vi "meb2cx_ver4_1_16bit.vi"() -> ()   [LabVIEW 2019]
uses:
  <vilib>/Analysis/3filter.llb/Filter Passband Type.ctl
  <vilib>/Utility/error.llb/DialogType.ctl
  <vilib>/DAQmx/write.llb/DAQmx Write (Analog 2D DBL NChan NSamp).vi
  <vilib>/DAQmx/read.llb/DAQmx Read (Analog 1D DBL 1Chan NSamp).vi
  <vilib>/DAQmx/read.llb/DAQmx Read (Analog 2D DBL NChan NSamp).vi
  <vilib>/Analysis/8numeric.llb/1D Numeric Integration.vi
  <vilib>/DAQmx/write.llb/DAQmx Write (Digital U16 1Chan 1Samp).vi
  <vilib>/DAQmx/read.llb/DAQmx Read (Analog DBL 1Chan 1Samp).vi
  <vilib>/Utility/file.llb/Read Delimited Spreadsheet (DBL).vi
  <vilib>/DAQmx/create/channels.llb/DAQmx Create Channel (DO-Digital Output).vi
  <vilib>/DAQmx/create/channels.llb/DAQmx Create Channel (AO-Voltage-Basic).vi
  <vilib>/DAQmx/create/channels.llb/DAQmx Create Channel (AI-Voltage-Basic).vi
  <vilib>/Analysis/3filter.llb/Butterworth Filter (DBL).vi
  <vilib>/DAQmx/configure/timing.llb/DAQmx Timing (Sample Clock).vi
  <vilib>/DAQmx/miscellaneous.llb/DAQmx Fill In Error Info.vi
  <vilib>/DAQmx/configure/trigger.llb/DAQmx Start Trigger (Digital Edge).vi
  <vilib>/Utility/file.llb/Write Delimited Spreadsheet (DBL).vi
  <vilib>/measure/madcrms.llb/Averaged DC-RMS for 1 Chan.vi
  <vilib>/measure/mascope.llb/Amplitude and Levels 1 chan.vi
  <vilib>/addons/Digital Filter Design/Process.llb/DFD Filtering (Array).vi
  <vilib>/Analysis/Matrix/Numeric/Conversions/Array To Matrix - RA2.vi
  <vilib>/Analysis/Matrix/Comparison/Equal/Equal - RM,RM.vi
  <vilib>/measure/NI_MAPro.lvlib
  <vilib>/Analysis/NI_AALPro.lvlib
  <vilib>/Analysis/NI_AAL_SigProc.lvlib
  <vilib>/Analysis/NI_AALBase.lvlib
  <resource>/objmgr/daqmx.rc
  <vilib>/gmath/NI_Gmath.lvlib
  <vilib>/addons/Digital Filter Design/NI_DigFilterLicensed.lvlib
  <vilib>/Analysis/Matrix/NI_Matrix.lvlib
panel:
  in  "stop delay":bool
  out "GERROR":bool
  out "error out 2":errorcluster
  out "error out":errorcluster
  out "CAL2":dbl[](array[numeric])
  out "YY":dbl[](array[numeric])
  out "XX":dbl[](array[numeric])
  out "F Si PSI":dbl format="%#.0f"
  out "bool_list":bool
  in  "Pomiar_main":bool
  out "Saveindi":bool=TRUE
  in  "Tab Control":enum32{"STAT", "MEAS", "CAL", "STOR", "TOOL"}(tab)
  out "Dev_Ready":bool
  out "Waveform Graph 5":dbl[][](graph)
  out "Bat_Low":bool
  out "Waveform Graph 4":dbl[][](graph)
  out "wz":u8[](array[numeric])=[0, 1, 2, 4, 5, 6, 8, 9, 10, 12, 13, 14, 28, 29, 30, 44, 45, 46, 60, 76, 77, 78, 92, 93, 94, 108, 109, 110, 124, 140, 141]
  in  "Gfreq":dbl=10.0 format="%0.4e"
  in  "stop":bool
  out "Supply [V]":dbl format="%#.1f"
  in  "Gain\n[dB]":u8 max=60 step=2
  in  "DEL":bool
  out "F Quality":dbl format="%#.0f"
  out "F Si":dbl format="%#.0f"
  in  "FREEZE":bool
  out "Si[MPa]":dbl max=200.0 format="%#.0f"
  out "Count":i32
  out "Waveform Graph 2":dbl[](graph)
  out "Low_L":dbl format="%.2g"
  out "Hi_L":dbl format="%.2g"
  out "AMP":dbl format="%.1f"
  out "INT":i32 format="%#.0f"
  out "XY Graph 2":cluster{"X":dbl, "Y":dbl}[](graph)
  in  "Oblicz":bool
  in  "SAVE":bool
  out "REC.":dbl
  out "Quality":i32
  out "F INT":dbl format="%#.0f"
  out "F Count":dbl
  out "F Amp":dbl format="%.1g"
  in  "AUTO":bool
  in  "Manual":bool
  in  "Delete cal file":bool
  out "Si [MPa]":dbl format="%#.0f"
  out "Int/Count":dbl format="%#.0f"
  out "cal3":dbl
  out "cal2":dbl
  out "cal1":dbl format="%#.0f"
  in  "OK cal3":bool
  in  "OK cal2":bool
  in  "OK cal1":bool
  out "XY Graph":cluster{"X":dbl, "Y":dbl}[](graph)
  in  "Load calibration":bool
  out "Quality":dbl format="%#.1f"
  in  "Calibration file to load":string(combo)
  in  "Import calibration files":bool
  out "cal4":dbl
  in  "OK cal4":bool
  in  "ListuDow":bool
  in  "Delete content":bool
  in  "Listbox":i32(listbox)=-1
  out "Active file":string
  out "Preview":dbl[](graph)
  in  "Save data file":bool
  in  "File load and\nexport source":string(combo)="A"
  in  "Export to drive":bool
  out "Export in\nprogress":bool
  in  "Preview data":bool
  in  "Delete folder content":bool
  in  "Plot selection":u16(ring) items=["AMP"=0, "INT"=3, "Count"=4, "Si[MPa]"=5, "Quality"=6]
  in  "ListUP":bool
  in  "FFT RANGE":i32 min=0
  in  "Update":bool
  in  "Set time":bool
  out "Waveform Graph 6":cluster{"rms_sign":dbl[]}[](graph)
  in  "filtrFFT":dbl=10.0 format="%0.2p"
  in  "filtrRMS":dbl=25.0 format="%0.2p"
  in  "THRESHOLD":dbl=1.7999999999999998 min=0.0 max=5.0 step=0.2
  in  "SOURCE":bool
  in  "FFT RANGE":cluster{"START":dbl, "END":dbl}[](array[cluster])
  out "XY Graph 3":cluster{"X":dbl, "Y":dbl}[](graph)
  out "Waveform Graph":cluster{"Filtered X":dbl[]}[](graph)
  in  "CF":dbl=5.000000000000002 min=0.0 max=10.0 step=0.2
  out "Waveform Graph 3":dbl[](graph)
  in  "Del_ZERO":bool
  in  "P_Zero":bool
  out "Boolean 8":bool
  out "Boolean 7":bool
  out "Boolean 6":bool
  out "Boolean 5":bool
  out "enUP":dbl format="%#.1g"
  out "Byłem":bool
  out "MPzero":dbl[][](array[numeric])
  out "Licznik":u8 max=60 step=2
  out "AAZero":dbl[][](array[numeric])
  out "P_Quality":i32
  out "TLO":dbl[](array[numeric])
  out "HBN_LOOP":dbl[](array[numeric])
  out "OK":bool
  out "Low_L 2":dbl format="%.2g"
  out "Hi_L 2":dbl format="%.2g"
  out "Data output":dbl[][](array[numeric])
  out "CAL":dbl[][](array[numeric])
  out "BAT":refnum<k21>
  out "ALL":dbl[][](array[numeric]) format="%0.2f"
  out "HBN":dbl[](array[numeric]) format="%0.2f"
  out "Trest":refnum<k21>
  out "Thbn":refnum<k21>
  out "Tgen":refnum<k21>
  out "Twz":refnum<k21>
  # "MAGSTRESS 5C - ser. 20200005"
  # "ver 4_1_16bit"
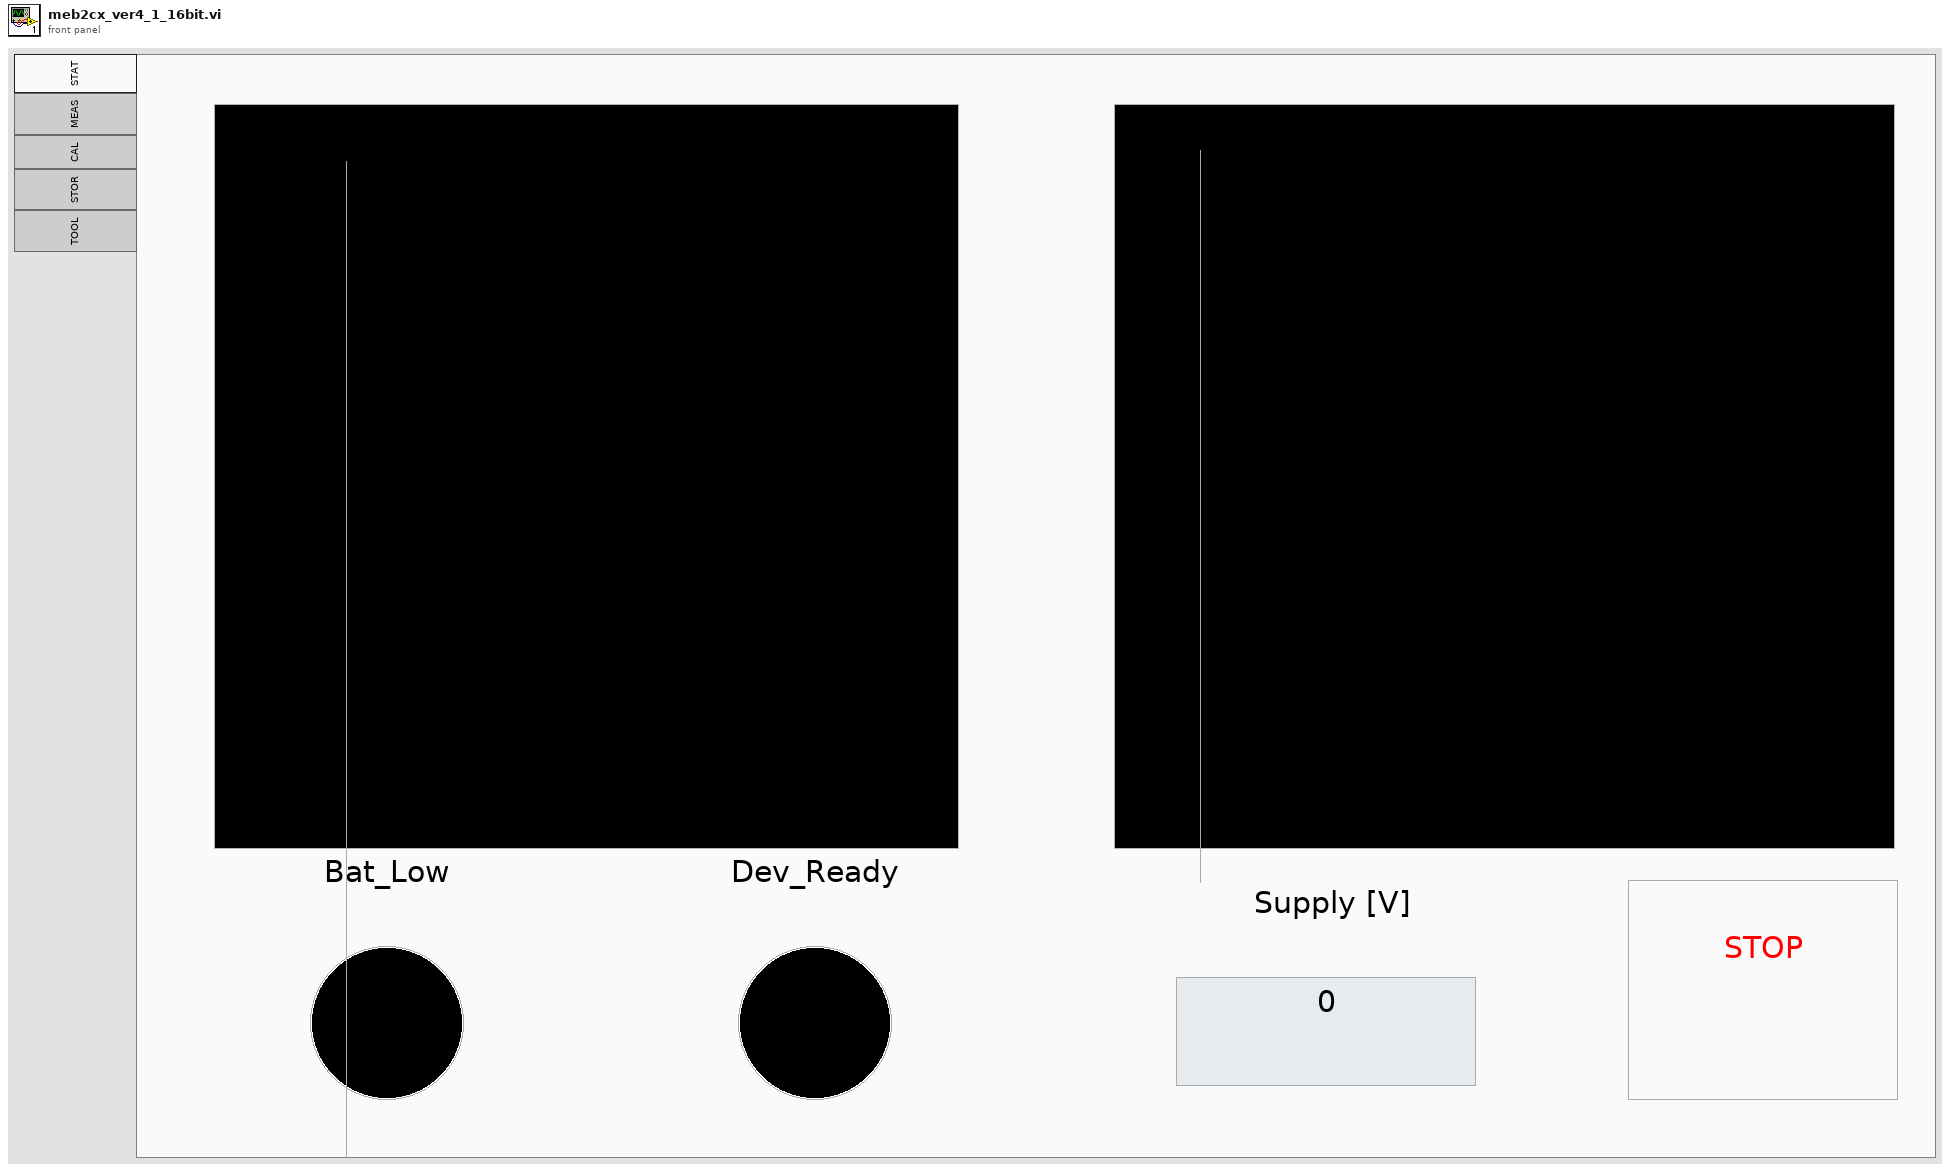
[diagram p1: front panel]
types:
  T1 = enum8{"Enabled", "Disabled", "Disabled and Grayed Out"}
  T2 = typedef "NI_AALBase.lvlib/Filter Passband Type.ctl" = enum32{"Lowpass", "Highpass", "Bandpass", "Bandstop"}
  T3 = typedef "DialogType.ctl" = u16
  T4 = typedef "NI_DigFilterLicensed.lvlib/DFD Filter Obj.ctl" = cluster{"mSRate_Fs":dbl, "mSRate_Version":string, "mSRate_Comments":string, "mSRate_OrgCoef":T5, "mSRate_CurCoef":T5, "mSRate_Quantized?":bool, "mSRate_QCoef":T5, "mSRate_QSettings":T7[], "mSRate_Order":i32, "mSRate_Scaling":cluster{"mSRate_ScaleByPowerOf2?":bool, "mSRate_ScaleType":T9}}
  T5 = typedef "NI_DigFilterLicensed.lvlib/DFD Filter Coef.ctl" = cluster{"type":T6, "gain":dbl, "coef a (k)":dbl[], "coef b (v)":dbl[]}
  T6 = typedef "NI_DigFilterLicensed.lvlib/DFD Filter Structure Type Selector.ctl" = enum16{"Undefined", "FIR Direct Form", "FIR Direct Form Transposed", "FIR Symmetric", "FIR Antisymmetric", "IIR Direct Form I", "IIR Direct Form I Transposed", "IIR Direct Form II", "IIR Direct Form II Transposed", "IIR Cascaded Second Order Sections Form I", "IIR Cascaded Second Order Sections Form I Transposed", "IIR Cascaded Second Order Sections Form II", "IIR Cascaded Second Order Sections Form II Transposed", "Lattice Allpass (basic sections)", "Lattice Allpass (one multiplier sections)", "Lattice Allpass (normalized sections)", "Lattice AR (basic sections)", "Lattice AR (one multiplier sections)", "Lattice AR (normalized sections)", "Lattice MA (minimum phase)", "Lattice MA (maximum phase)", "Lattice ARMA (basic sections)", "Lattice ARMA (one multiplier sections)", "Lattice ARMA (normalized sections)"}
  T7 = typedef "NI_DigFilterLicensed.lvlib/dfd_Internal Quantization Settings.ctl" = cluster{"source":T8, "wl":i16, "iwl":i16, "overflow mode":enum16{"Saturation", "Wrap"}, "rounding mode":enum16{"Nearest", "Truncation"}, "signed?":bool}
  T8 = typedef "NI_DigFilterLicensed.lvlib/dfd_Internal Quantization Srcs.ctl" = u16
  T9 = typedef "NI_DigFilterLicensed.lvlib/DFD Coef Norm Type.ctl" = enum16{"No Norm", "Time Domain 1-Norm", "Time Domain 2-Norm", "Time Domain Inf-Norm"}
  T10 = typedef "NI_Matrix.lvlib/RealMatrix.ctl" = dbl[][]
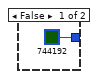
[diagram p3: hidden frame]
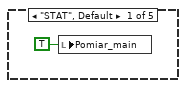
[diagram p4: hidden frame]
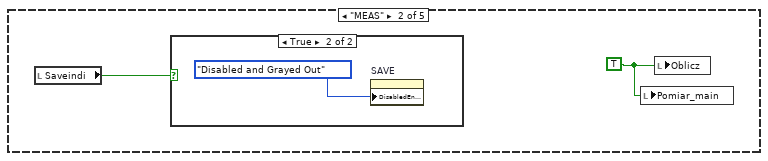
[diagram p5: hidden frame]
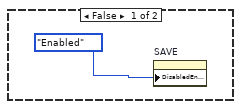
[diagram p6: hidden frame]
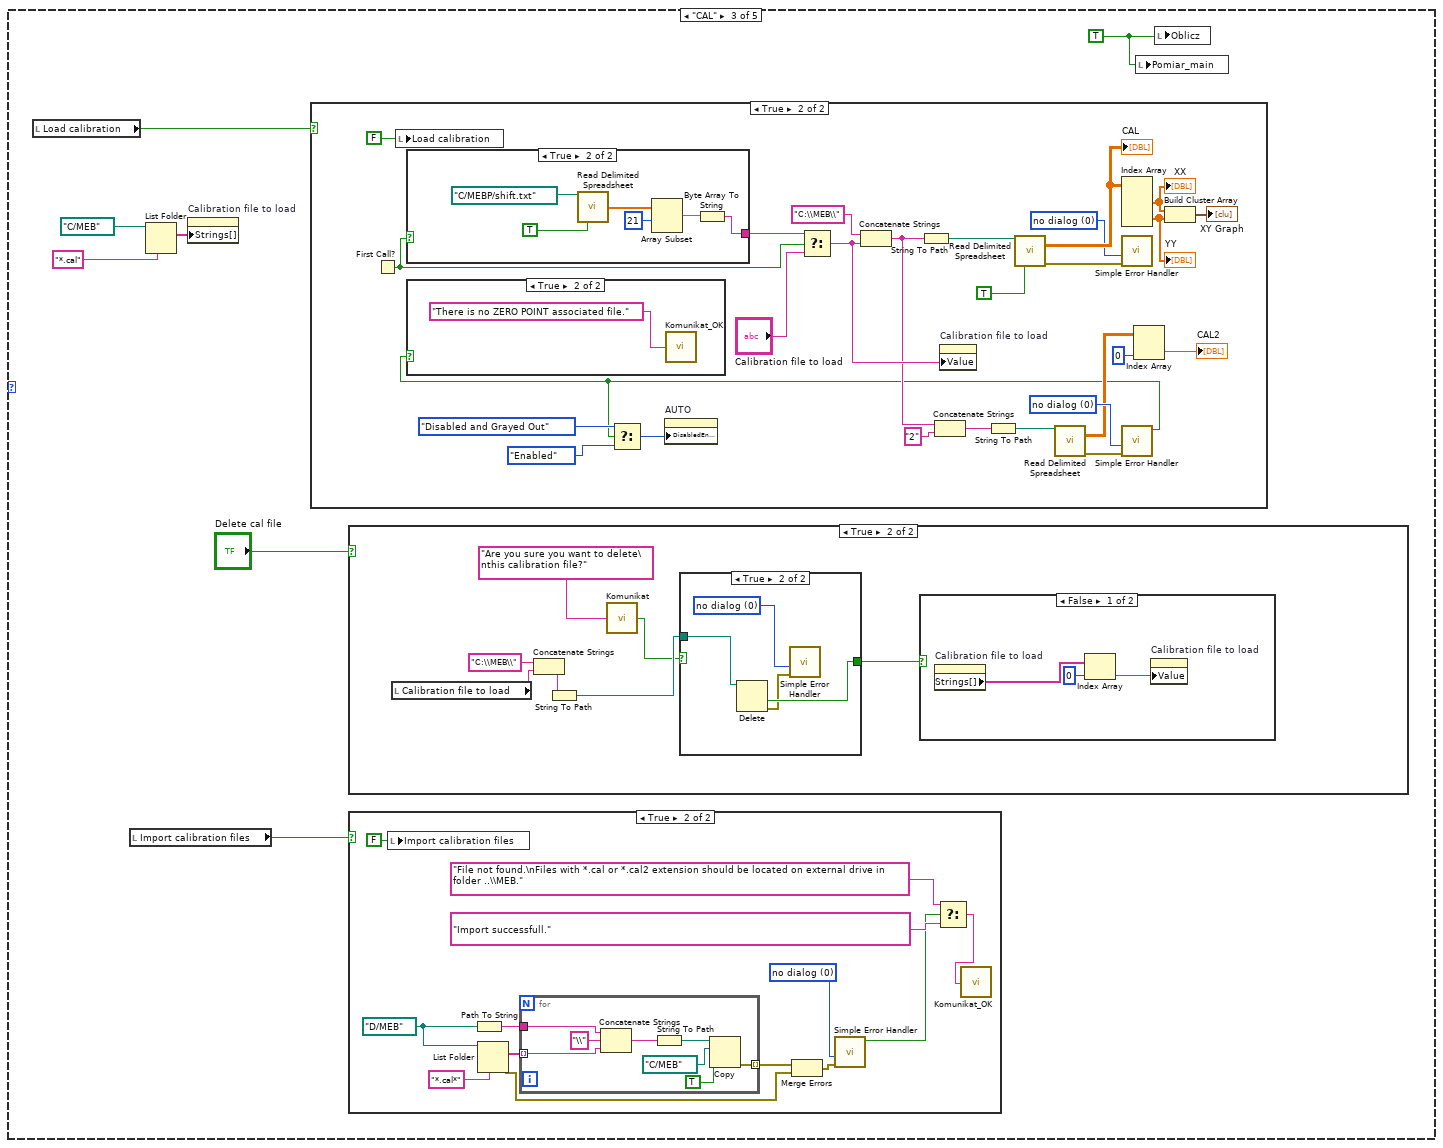
[diagram p7: hidden frame]
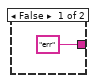
[diagram p14: hidden frame]
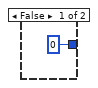
[diagram p16: hidden frame]
diagram:
  n1 = flat-sequence {
    frame #0 {
      n2 = flat-sequence {
        frame #0 {
          w28 = TRUE
          n3 = call-poly <vilib>:"Read Delimited Spreadsheet.vi"("file path (dialog if empty)"=path "C:/MEBP/shift.txt", "transpose? (F)"=TRUE) -> ("first row"=w26:dbl[])  [unwired: 8 in, 5 out]
          n4 = Array Subset(array=w26, index=7, length=14) -> (w23:dbl[])
          n5 = Index Array(array=w23) -> (element #1=w22:dbl, element #2=w21:dbl, element #3=w20:dbl, element #4=w19:dbl, element #5=w18:dbl, element #6=w17:dbl, element #7=w16:dbl, element #8=w15:dbl, element #9=w9:dbl, element #10=w8:dbl, element #11=w7:dbl, element #12=w6:dbl, element #13=w5:dbl, element #14=w4:dbl)  [unwired: 14 in]
          n6 = Bundle("Numeric"=w22, "Numeric"=w21) -> (w14:cluster{"Numeric":dbl, "Numeric":dbl})  [unwired: 1 in]
          n7 = Bundle("Numeric"=w20, "Numeric"=w19) -> (w13:cluster{"Numeric":dbl, "Numeric":dbl})  [unwired: 1 in]
          n8 = Bundle("Numeric"=w18, "Numeric"=w17) -> (w12:cluster{"Numeric":dbl, "Numeric":dbl})  [unwired: 1 in]
          n9 = Bundle("Numeric"=w16, "Numeric"=w15) -> (w11:cluster{"Numeric":dbl, "Numeric":dbl})  [unwired: 1 in]
          n10 = Bundle("Numeric"=w9, "Numeric"=w8) -> (w3:cluster{"Numeric":dbl, "Numeric":dbl})  [unwired: 1 in]
          n11 = Bundle("Numeric"=w7, "Numeric"=w6) -> (w2:cluster{"Numeric":dbl, "Numeric":dbl})  [unwired: 1 in]
          n12 = Bundle("Numeric"=w5, "Numeric"=w4) -> (w1:cluster{"Numeric":dbl, "Numeric":dbl})  [unwired: 1 in]
          n13 = Build Array(w14, w13, w12, w11, w3, w2, w1) -> (w10:cluster{"Numeric":dbl, "Numeric":dbl}[])
          n14 = local write "FFT RANGE"(w10) -> ()
          n15 = Index Array(array=w26) -> (element #1=w35:dbl, element #2=w34:dbl, element #3=w33:dbl, element #4=w32:dbl, element #5=w31:dbl, element #6=w30:dbl, element #7=w29:dbl)  [unwired: 7 in]
          n16 = local write "Load calibration"(w28) -> ()
          n17 = local write "Gain\n[dB]"(w35) -> ()
          n18 = local write "cal1"(w34) -> ()
          n19 = local write "cal2"(w33) -> ()
          n20 = local write "cal3"(w32) -> ()
          n21 = local write "cal4"(w31) -> ()
          n22 = local write "THRESHOLD"(w30) -> ()
          n23 = local write "CF"(w29) -> ()
          n24 = call-poly <vilib>:"Read Delimited Spreadsheet.vi"("file path (dialog if empty)"=path "C:/MEBP/pzero.txt") -> ("all rows"=→"MPzero":dbl[][])  [unwired: 9 in, 5 out]
          n25 = local write "OK cal1"(w28) -> ()
          n26 = local write "OK cal2"(w28) -> ()
          n27 = local write "OK cal3"(w28) -> ()
          n28 = local write "OK cal4"(w28) -> ()
        }
        frame #1 {
          n29 = while {
            i -> [w42]
            stop <- w45 continue-if-true
            n30 = Equal?(x=w42, y=10 ("x")) -> (x = y?=w40:bool)
            n31 = call <vilib>:"DAQmx Self-Test Device.vi"("device in"=tag "Dev1") -> ("error out"=w45:errorcluster)  [unwired: 14 in]
            n32 = Unbundle By Name(w45) -> ("status"=w43:bool)
            n33 = And(x=w40, y=w43) -> (x .and. y?=w39:bool)
            n34 = case shown="True" w39 {
              frame False {
              }
              frame True {
                n35 = flat-sequence {
                  tunnel: path "C:/ProgramData/National Instruments/MAX" ("target path (use dialog)") -> [w51]
                  frame #0 {
                    n36 = call <vilib>:"System Exec.vi"("run minimized? (F)"=FALSE ("wait until completion? (T)"), "wait until completion? (T)"=TRUE, "command line"="cmd /r \"mx.lnk\"") -> ()  [unwired: 5 in, 4 out]
                  }
                  frame #1 {
                    n37 = Copy(9:TRUE ("overwrite (F)"), 10:w51, 11:path "C:/MEBP/MAX" ("source path")) -> ()  [unwired: 2 in, 3 out]
                  }
                  frame #2 {
                    n38 = call <vilib>:"System Exec.vi"("run minimized? (F)"=FALSE ("wait until completion? (T)"), "wait until completion? (T)"=TRUE, "command line"="cmd /r \"mxs.lnk\"") -> ()  [unwired: 5 in, 4 out]
                  }
                }
              }
            }
            n39 = Not(x=w43) -> (.not. x?=→"Dev_Ready":bool)
          }
        }
        frame #2 {
          w59 = 0.0 ("F Amp")
          w72 = 10083 items=["Default"=-1, "RSE"=10083, "NRSE"=10078, "Differential"=10106, "Pseudodifferential"=12529] ("input terminal configuration")
          w77 = 10083 items=["Default"=-1, "RSE"=10083, "NRSE"=10078, "Differential"=10106, "Pseudodifferential"=12529] ("input terminal configuration")
          w82 = 10083 items=["Default"=-1, "RSE"=10083, "NRSE"=10078, "Differential"=10106, "Pseudodifferential"=12529] ("input terminal configuration")
          w86 = 10083 items=["Default"=-1, "RSE"=10083, "Differential"=10106, "Pseudodifferential"=12529] ("output terminal configuration")
          # "...i nadanie im rozmiaru"
          # "Wybór wszystkich elementów listboxa..."
          n40 = Initialize Array(0.0 ("element"), 400 ("dimension size")) -> (→"TLO" →"HBN_LOOP":dbl[])
          n41 = property on="Listbox" class="LstBox (strict)"("Active Row"=-2 ("Active Row:Active Row Number")) -> ()  [unwired: 2 in, 2 out]
          n42 = property on="Listbox" class="LstBox (strict)"("CellFontSize"=u32 70 ("Active Row:Cell Font:Size")) -> ()  [unwired: 2 in, 2 out]
          n43 = Initialize Array(0.0 ("element")) -> (→"AAZero":dbl[][])  [unwired: 2 in]
          n44 = local write "enUP"(w59) -> ()
          n45 = call-poly <vilib>:"DAQmx Create Virtual Channel.vi"("lines"=tag "Dev1/port0/line0:15") -> ("task out"=→"Twz":refnum<k21>)  [unwired: 13 in, 1 out]
          n46 = local write "Saveindi"(TRUE ("Saveindi")) -> ()
          n47 = call-poly <vilib>:"DAQmx Create Virtual Channel.vi"("maximum value"=10.0, "minimum value"=-10.0, "input terminal configuration"=w72, "physical channels"=tag "Dev1/ai4") -> ("task out"=→"BAT":refnum<k21>)  [unwired: 10 in, 1 out]
          n48 = property on="stop" class="Bool (strict)"("DisabledEnum"=T1."Enabled" ("Disabled")) -> ()  [unwired: 2 in, 2 out]
          n49 = property on="File load and\nexport source" class="CmbBox"("Text.FontSize"=u32 100 ("Text.Font:Size")) -> ()  [unwired: 2 in, 2 out]
          n50 = call-poly <vilib>:"DAQmx Create Virtual Channel.vi"("maximum value"=10.0, "minimum value"=-10.0, "input terminal configuration"=w82, "physical channels"=tag "Dev1/ai0") -> ("task out"=→"Thbn":refnum<k21>)  [unwired: 10 in, 1 out]
          n51 = call-poly <vilib>:"DAQmx Create Virtual Channel.vi"("maximum value"=10.0, "minimum value"=-10.0, "output terminal configuration"=w86, "physical channels"=tag "Dev1/ao0:1") -> ("task out"=→"Tgen":refnum<k21>)  [unwired: 10 in, 1 out]
          n52 = call-poly <vilib>:"DAQmx Create Virtual Channel.vi"("maximum value"=10.0, "minimum value"=-10.0, "input terminal configuration"=w77, "physical channels"=tag "Dev1/ai1:3") -> ("task out"=→"Trest":refnum<k21>)  [unwired: 10 in, 1 out]
          "wz" <- u8[] [0, 1, 2, 4, 5, 6, 8, 9, 10, 12, 13, 14, 28, 29, 30, 44, 45, 46, 60, 76, 77, 78, 92, 93, 94, 108, 109, 110, 124, 140, 141]
          "F Amp" <- w59
          "Hi_L 2" <- w59
          "Low_L 2" <- w59
          "F INT" <- w59
          "F Count" <- w59
          "F Si" <- w59
          "Licznik" <- u8 0 ("Licznik")
          "Byłem" <- TRUE ("Byłem")
          "F Quality" <- w59
          "F Si PSI" <- w59
        }
      }
    }
    frame #1 {
      w123 = 200000 ("Gsamples")
      w118 = 10097 items=["Allow Regeneration"=10097, "Do Not Allow Regeneration"=10158] ("RegenMode")
      w121 = 10123 items=["Finite Samples"=10178, "Continuous Samples"=10123, "Hardware Timed Single Point"=12522] ("sample mode")
      # "Generator"
      n53 = Reciprocal(x=500000.0) -> (1/x=w102:dbl)
      n54 = Multiply(x=w102, y="Gfreq") -> (x*y=w97:dbl)
      n55 = Divide(x=w97, y=6.0) -> (x/y=w96:dbl)
      n56 = local read "Tgen"() -> (w114:refnum<k21>)
      n57 = call <vilib>:"Triangle Wave.vi"("samples"=w123, "amplitude"=4.5 ("Gamp"), "frequency"=w97, "phase in"=0.0) -> ("triangle wave"=w94:dbl[])  [unwired: 1 in, 2 out]
      n58 = call <vilib>:"Square Wave.vi"("samples"=w123, "amplitude"=2.5, "frequency"=w96, "duty cycle (%)"=50.0, "phase in"=163.0) -> ("square wave"=w105:dbl[])  [unwired: 1 in, 2 out]
      n59 = call <vilib>:"DAQmx Stop Task.vi"("task/channels in"=w114) -> ("task out"=w113:refnum<k21>, "error out"=w112:errorcluster)  [unwired: 13 in]
      n60 = call-poly <vilib>:"Butterworth Filter.vi"("order"=4, "filter type"=Filter_Passband_Type."Lowpass", "low cutoff freq: fl"=0.001, "sampling freq: fs"=1.0, "X"=w94) -> ("Filtered X"=w93:dbl[])  [unwired: 3 in, 1 out]
      n61 = call-poly <vilib>:"DAQmx Timing.vi"("task/channels in"=w113, "sample mode"=w121, "samples per channel"=w123, "rate"=500000.0, "error in"=w112) -> ("task out"=w120:refnum<k21>)  [unwired: 9 in, 1 out]
      n62 = Add(x=w105, y=2.5) -> (x+y=w104:dbl[])
      n63 = property class="DAQmx Write"(reference=w120, "Regeneration Mode"=w118) -> (reference out=w119:refnum<k21>)  [unwired: 1 in, 1 out]
      n64 = Build Array(w93, w104) -> (w95:dbl[][])
      "Waveform Graph 4" <- w95
      n65 = call-poly <vilib>:"DAQmx Write.vi"("task/channels in"=w119, "auto start"=FALSE, "data"=w95) -> ("task out"=w116:refnum<k21>, "error out"=w115:errorcluster)  [unwired: 10 in, 1 out]
      n66 = call <vilib>:"DAQmx Start Task.vi"("task/channels in"=w116, "error in"=w115) -> ()  [unwired: 12 in, 2 out]
    }
    frame #2 {
      n67 = Initialize Array(0.0 ("element")) -> (w126:dbl[][])  [unwired: 2 in]
      n68 = while {
        shift-right: [w146] -> _
        shift-left: w126 -> [w132]
        stop <- FALSE stop-if-true
        n69 = flat-sequence {
          tunnel: w132 -> [w443]
          tunnel: [w443] -> w131
          tunnel: w131 -> [w698]
          tunnel: [w705] -> w130
          tunnel: [w704] -> w129
          frame #0 {
            n70 = Or(x="Pomiar_main", y="Save data file") -> (x .or. y?=w440:bool)
            n71 = case shown="True" w440 {
              tunnel: [FALSE ("GERROR 2") w445] -> w439
              frame False {
                (unwired) TRUE ("Save data file")
              }
              frame True {
                n72 = flat-sequence {
                  tunnel: [w447] -> w446
                  tunnel: w446 -> [w468]
                  tunnel: [w466] -> w445
                  frame #0 {
                    w448 = T3 0 items=["no dialog", "OK message", "continue or stop message", "OK message + warnings", "continue/stop + warnings"] ("type of dialog (OK msg:1)")
                    w455 = 10171 items=["Rising"=10280, "Falling"=10171] ("edge")
                    w461 = 10280 items=["Rising"=10280, "Falling"=10171] ("active edge")
                    w451 = 400000.0 ("rate")
                    w463 = 10178 items=["Finite Samples"=10178, "Continuous Samples"=10123, "Hardware Timed Single Point"=12522] ("sample mode")
                    # "Pomiar Główny"
                    n73 = local read "Gfreq"() -> (w462:dbl)
                    n74 = Divide(x=w451, y=w462) -> (x/y=w453:dbl)
                    n75 = Multiply(x=3.0, y=w453) -> (x*y=w452:dbl)
                    n76 = local read "Thbn"() -> (w464:refnum<k21>)
                    n77 = call-poly <vilib>:"DAQmx Timing.vi"("task/channels in"=w464, "sample mode"=w463, "samples per channel"=w452, "rate"=w451, "active edge"=w461) -> ("task out"=w460:refnum<k21>, "error out"=w457:errorcluster)  [unwired: 9 in]
                    n78 = call-poly <vilib>:"DAQmx Trigger.vi"("task/channels in"=w460, "source"=tag "/Dev1/PFI0", "edge"=w455, "error in"=w457) -> ("task out"=w459:refnum<k21>, "error out"=w458:errorcluster)  [unwired: 10 in]
                    n79 = call-poly <vilib>:"DAQmx Read.vi"("task/channels in"=w459, "number of samples per channel"=w452, "error in"=w458) -> ("data"=→"HBN":dbl[], "error out"=w449:errorcluster)  [unwired: 10 in, 1 out]
                    n80 = call <vilib>:"Simple Error Handler.vi"("type of dialog (OK msg:1)"=w448, "error in (no error)"=w449) -> ("error?"=w447:bool)  [unwired: 3 in, 4 out]
                  }
                  frame #1 {
                    w470 = T3 0 items=["no dialog", "OK message", "continue or stop message", "OK message + warnings", "continue/stop + warnings"] ("type of dialog (OK msg:1)")
                    w485 = 10171 items=["Rising"=10280, "Falling"=10171] ("edge")
                    w479 = 10280 items=["Rising"=10280, "Falling"=10171] ("active edge")
                    w477 = 100000.0 ("rate")
                    w476 = 10178 items=["Finite Samples"=10178, "Continuous Samples"=10123, "Hardware Timed Single Point"=12522] ("sample mode")
                    # "Pomiar pozstały \"rzadki\""
                    # "Pomiar pozostały \"rzadki\""
                    n81 = local read "Gfreq"() -> (w478:dbl)
                    n82 = Divide(x=w477, y=w478) -> (x/y=w473:dbl)
                    n83 = Multiply(x=1.0, y=w473) -> (x*y=w472:dbl)
                    n84 = local read "Trest"() -> (w475:refnum<k21>)
                    n85 = call-poly <vilib>:"DAQmx Timing.vi"("task/channels in"=w475, "sample mode"=w476, "samples per channel"=w472, "rate"=w477, "active edge"=w479) -> ("task out"=w480:refnum<k21>, "error out"=w483:errorcluster)  [unwired: 9 in]
                    n86 = call-poly <vilib>:"DAQmx Trigger.vi"("task/channels in"=w480, "source"=tag "/Dev1/PFI0", "edge"=w485, "error in"=w483) -> ("task out"=w481:refnum<k21>, "error out"=w482:errorcluster)  [unwired: 10 in]
                    n87 = call-poly <vilib>:"DAQmx Read.vi"("task/channels in"=w481, "number of samples per channel"=w472, "error in"=w482) -> ("data"=→"ALL" →"Waveform Graph 5":dbl[][], "error out"=w469:errorcluster)  [unwired: 10 in, 1 out]
                    n88 = call <vilib>:"Simple Error Handler.vi"("type of dialog (OK msg:1)"=w470, "error in (no error)"=w469) -> ("error?"=w467:bool)  [unwired: 3 in, 4 out]
                    n89 = Or(x=w468, y=w467) -> (x .or. y?=w466:bool)
                    n90 = case shown="True" w466 {
                      tunnel: [FALSE w487] -> w465
                      frame False {
                      }
                      frame True {
                        n91 = feedback #1(0.0) -> (w491:dbl)
                        n92 = Increment(x=w491) -> (x+1=w489:dbl)
                        n93 = feedback-in #1(w489) -> ()
                        n94 = Equal?(x=w489, y=2.0) -> (x = y?=w487:bool)
                      }
                    }
                    n95 = case shown="True" w465 {
                      frame False {
                      }
                      frame True {
                        n96 = local read "Calibration file to load"() -> (w521:string)
                        n97 = local read "THRESHOLD"() -> (w524:dbl)
                        n98 = local read "Gain\n[dB]"() -> (w529:u8)
                        n99 = local read "cal1"() -> (w528:dbl)
                        n100 = local read "cal2"() -> (w527:dbl)
                        n101 = local read "cal3"() -> (w526:dbl)
                        n102 = local read "cal4"() -> (w525:dbl)
                        n103 = local read "CF"() -> (w523:dbl)
                        n104 = String To Byte Array(string=w521) -> (unsigned byte array=w504:u8[])
                        n105 = call "Komunikat_OK.vi"("String 2"="Measurement Error.\nThe device will be shut down in 20 seconds." ("message")) -> ()  [unwired: 1 out]
                        n106 = local read "FFT RANGE"() -> (w503:cluster{"START":dbl, "END":dbl}[])
                        n107 = Index Array(array=w503) -> (element #1=w508:cluster{"START":dbl, "END":dbl}, element #2=w505:cluster{"START":dbl, "END":dbl}, element #3=w506:cluster{"START":dbl, "END":dbl}, element #4=w507:cluster{"START":dbl, "END":dbl}, element #5=w495:cluster{"START":dbl, "END":dbl}, element #6=w494:cluster{"START":dbl, "END":dbl}, element #7=w493:cluster{"START":dbl, "END":dbl})  [unwired: 7 in]
                        n108 = Unbundle(w508) -> ("START"=w509:dbl, "END"=w510:dbl)
                        n109 = Unbundle(w505) -> ("START"=w511:dbl, "END"=w512:dbl)
                        n110 = Unbundle(w506) -> ("START"=w513:dbl, "END"=w514:dbl)
                        n111 = Unbundle(w507) -> ("START"=w515:dbl, "END"=w516:dbl)
                        n112 = Unbundle(w495) -> ("START"=w501:dbl, "END"=w500:dbl)
                        n113 = Unbundle(w494) -> ("START"=w499:dbl, "END"=w498:dbl)
                        n114 = Unbundle(w493) -> ("START"=w497:dbl, "END"=w496:dbl)
                        n115 = Build Array(w509, w510, w511, w512, w513, w514, w515, w516, w501, w500, w499, w498, w497, w496) -> (w502:dbl[])
                        n116 = Build Array (concatenate)(w529, w528, w527, w526, w525, w524, w523, w502, w504) -> (w522:dbl[])
                        n117 = call-poly <vilib>:"Write Delimited Spreadsheet.vi"("file path (dialog if empty)"=path "C:/MEBP/shift.txt", "format (%.3f)"="%.0", "1D data"=w522, "append to file? (new file:F)"=FALSE) -> ()  [unwired: 10 in, 2 out]
                        n118 = call <vilib>:"System Exec.vi"("command line"="shutdown -s -f -t 20") -> ()  [unwired: 7 in, 4 out]
                      }
                    }
                  }
                  frame #2 {
                    n119 = flat-sequence {
                      frame #0 {
                        # "Obliczenie jednoosiowe"
                        n120 = flat-sequence {
                          frame #0 {
                            n121 = local read "SOURCE"() -> (w532:bool)
                            n122 = local read "Count"() -> (w530:i32)
                            n123 = local read "INT"() -> (w531:i32)
                            n124 = Select(t=w530, s=w532, f=w531) -> (s? t:f=→"Int/Count":i32)
                          }
                          frame #1 {
                            w543 = 1 items=["nearest", "linear", "spline", "cubic Hermite", "Lagrange"] ("method")
                            n125 = local read "Quality"() -> (→"Quality":i32)
                            n126 = local read "cal1"() -> (w557:dbl)
                            n127 = local read "cal2"() -> (w558:dbl)
                            n128 = local read "cal3"() -> (w559:dbl)
                            n129 = local read "cal4"() -> (w544:dbl)
                            n130 = Compound Arithmetic op=ADD(w557, w558, w559, w544) -> (w560:dbl)
                            n131 = local read "Int/Count"() -> (w555:dbl)
                            n132 = Divide(x=w560, y=4.0) -> (x/y=w554:dbl)
                            n133 = Divide(x=w555, y=w554) -> (x/y=w540:dbl)
                            n134 = Multiply(x=1.0, y=w540) -> (x*y=w551:dbl)
                            n135 = Multiply(x=1.0, y=w540) -> (x*y=w549:dbl)
                            n136 = Build Array(w551, w549) -> (w553:dbl[])
                            n137 = local read "YY"() -> (w542:dbl[])
                            n138 = local read "XX"() -> (w541:dbl[])
                            n139 = call <vilib>:"Interpolate 1D.vi"("method"=w543, "xi"=w553, "X"=w541, "Y"=w542) -> ("yi"=w548:dbl[])  [unwired: 5 in, 2 out]
                            n140 = Index Array(array=w548) -> (element #1=w547:dbl)  [unwired: 2 in, 1 out]
                            n141 = Multiply(x=w547, y=0.22) -> (x*y=w534:dbl)
                            n142 = Absolute Value(x=w534) -> (abs(x)=w539:dbl)
                            n143 = Greater?(x=w539, y=2000.0) -> (0:w537:bool)
                            n144 = Select(t=nan, s=w537, f=w534) -> (s? t:f=→"Si [MPa]" →"Si[MPa]":dbl)
                          }
                        }
                      }
                      frame #1 {
                        n145 = case shown="True" "Oblicz" {
                          frame False {
                          }
                          frame True {
                            n146 = flat-sequence {
                              frame #0 {
                                # "Blok Główny"
                                n147 = local read "HBN"() -> (w679:dbl[])
                                n148 = Build Array("FFT RANGE") -> (w601:i32[])
                                n149 = call "FIltrFFT_wielopasmowy.vi"("zakresy"="FFT RANGE", "f_sampl [kHz]"=400, "dane"=w679) -> ("FFTcut"=w673:cdb[], "FFT"=w674:cdb[], "sign_filtered"=w652:dbl[])  [unwired: 5 in, 1 out]
                                n150 = property on="FFT RANGE" class="Arr (strict)"("Index Values"=w601) -> ()  [unwired: 2 in, 2 out]
                                n151 = call-poly <vilib>:"Averaged DC-RMS.vi"("averaging time"=4.0, "signal in"=w652) -> ("DC value waveform"=w676:waveform(dbl))  [unwired: 5 in, 4 out]
                                n152 = call "myRMS.vi"("LptRMS"="filtrFFT", "dane"=w673) -> ("rms_sign"=w658:dbl[])  [unwired: 9 in]
                                n153 = call "myRMS.vi"("LptRMS"="filtrFFT", "dane"=w674) -> ("rms_sign"=w659:dbl[])  [unwired: 9 in]
                                n154 = local read "ALL"() -> (w677:dbl[][])
                                n155 = call <vilib>:"Peak Detector.vi"("width"=3, "threshold"="THRESHOLD", "X"=w652) -> ("# found"=→"Count":i32)  [unwired: 4 in, 4 out]
                                n156 = Array Subset(array=w652, index=0, length=40000) -> (→"Waveform Graph 2" →"Waveform Graph 3":dbl[])
                                n157 = Divide(x=100000.0, y="filtrRMS") -> (x/y=w667:dbl)
                                n158 = Build Cluster Array(w658, w659) -> (→"Waveform Graph 6":cluster{"rms_sign":dbl[]}[])
                                n159 = Unbundle By Name(w676) -> ("Y"=w675:dbl[])
                                n160 = Index Array(array=w677) -> (element #1=w671:dbl[], element #3=w604:dbl[])  [unwired: 6 in, 1 out]
                                n161 = Divide(x=9999 ("index"), y="filtrRMS") -> (x/y=w639:dbl)
                                n162 = Divide(x=19999 ("index"), y="filtrRMS") -> (x/y=w637:dbl)
                                n163 = Divide(x=10000 ("length"), y="filtrRMS") -> (x/y=w641:dbl)
                                n164 = call-poly <vilib>:"Averaged DC-RMS.vi"("averaging time"="filtrRMS", "signal in"=w671) -> ("DC value waveform"=w670:waveform(dbl))  [unwired: 5 in, 4 out]
                                n165 = Multiply(x=1.15, y=w604) -> (x*y=w603:dbl[])
                                n166 = call-poly <vilib>:"Amplitude and Levels.vi"("signal in"=w603) -> ("error out"=→"error out":errorcluster, "amplitude"=w654:dbl)  [unwired: 7 in, 2 out]
                                n167 = call "myRMS.vi"("LptRMS"="filtrRMS", "dane"=w675) -> ("rms_sign"=w649:dbl[])  [unwired: 9 in]
                                n168 = First Call?() -> (First Call?: T/F=w627:bool)
                                n169 = local read "Gain\n[dB]"() -> (w624:u8)
                                n170 = Array Subset(array=w649, index=w639, length=w641) -> (w646:dbl[])
                                n171 = Array Subset(array=w649, index=w637, length=w641) -> (w645:dbl[])
                                n172 = Multiply(x=w654, y=100.0) -> (x*y=w626:dbl)
                                "Quality" <- w626
                                n173 = case shown="True" w627 {
                                tunnel: w626 -> [_ w682]
                                frame False {
                                }
                                frame True {
                                n174 = local write "P_Quality"(w682) -> ()
                                }
                                }
                                n175 = local read "P_Quality"() -> (w631:i32)
                                n176 = Array Subset(array=w649, index=0, length=w641) -> (w647:dbl[])
                                n177 = Divide(x=w624, y=u8 2) -> (x/y=w622:dbl)
                                n178 = local read "MPzero"() -> (w625:dbl[][])
                                n179 = To Long Integer(number=w622) -> (32bit integer=w608:i32)
                                n180 = Subtract(x=w626, y=w631) -> (x-y=w633:dbl)
                                n181 = Compound Arithmetic op=ADD(w647, w646, w645) -> (w643:dbl[])
                                n182 = local read "Del_ZERO"() -> (w620:bool)
                                n183 = Index Array(array=w625, index (row)=w608) -> (element=w618:dbl[])  [unwired: 1 in]
                                n184 = Divide(x=w643, y=3.0) -> (x/y=w611:dbl[])
                                n185 = call "Butterworth Lowpass Filter"() -> ("filter out"=w612:T4)  [unwired: 10 in, 1 out]
                                n186 = local read "TLO"() -> (w619:dbl[])
                                n187 = Reciprocal(x=w667) -> (1/x=w666:dbl)
                                n188 = Divide(x="CF", y=1000.0) -> (x/y=w613:dbl)
                                n189 = Multiply(x=w633, y=w613) -> (x*y=w632:dbl)
                                n190 = Select(t=w619, s=w620, f=w618) -> (s? t:f=w621:dbl[])
                                n191 = Add(x=w632, y=1.0) -> (x+y=w629:dbl)
                                n192 = call-poly <vilib>:"DFD Filtering.vi"("init? (F)"=FALSE, "filter"=w612, "signal in"=w611) -> ("signal out"=w610:dbl[])  [unwired: 7 in, 1 out]
                                n193 = Compound Arithmetic op=MULTIPLY(w621, w629) -> (w616:dbl[])
                                n194 = local write "HBN_LOOP"(w610) -> ()
                                n195 = Build Cluster Array(w610, w616) -> (→"Waveform Graph":cluster{"signal out":dbl[]}[])
                                n196 = Unbundle By Name(w670) -> ("Y"=w669:dbl[])
                                n197 = Subtract(x=w610, y=w616) -> (x-y=w634:dbl[])
                                n198 = call-poly <vilib>:"Numeric Integration.vi"("dt"="filtrRMS", "Input Array"=w634) -> ("result"=→"INT":dbl)  [unwired: 1 in, 1 out]
                                n199 = Bundle By Name("dt"=w666, "Y"=w634) -> (w665:waveform(dbl))  [unwired: 1 in]
                                n200 = Build Cluster Array(w669, w634) -> (→"XY Graph 2" →"XY Graph 3":cluster{dbl, dbl}[])
                                n201 = call-poly <vilib>:"Amplitude and Levels.vi"("signal in"=w665) -> ("error out"=→"error out 2":errorcluster, "low state level"=→"Low_L":dbl, "high state level"=→"Hi_L":dbl, "amplitude"=→"AMP":dbl)  [unwired: 7 in]
                              }
                              frame #1 {
                                n202 = local write "Oblicz"(FALSE ("Oblicz")) -> ()
                              }
                            }
                          }
                        }
                        n203 = case shown="False" "OK cal1" {
                          tunnel: [0 w600] -> w566
                          frame True {
                          }
                          frame False {
                            n204 = local read "Count"() -> (w596:i32)
                            n205 = local read "SOURCE"() -> (w598:bool)
                            n206 = local read "INT"() -> (w597:i32)
                            n207 = property on="cal1" class="DigNum (strict)"() -> ("NumText.BGColor"=w600:u32)  [unwired: 2 in, 2 out]
                            n208 = Select(t=w596, s=w598, f=w597) -> (s? t:f=→"cal1":i32)
                          }
                        }
                        n209 = case shown="False" "OK cal2" {
                          tunnel: [0 w594] -> w565
                          frame True {
                          }
                          frame False {
                            n210 = local read "Count"() -> (w590:i32)
                            n211 = local read "SOURCE"() -> (w592:bool)
                            n212 = local read "INT"() -> (w591:i32)
                            n213 = property on="cal2" class="DigNum (strict)"() -> ("NumText.BGColor"=w594:u32)  [unwired: 2 in, 2 out]
                            n214 = Select(t=w590, s=w592, f=w591) -> (s? t:f=→"cal2":i32)
                          }
                        }
                        n215 = property on="cal1" class="DigNum (strict)"("NumText.TextColor"=w566) -> ()  [unwired: 2 in, 2 out]
                        n216 = property on="cal2" class="DigNum (strict)"("NumText.TextColor"=w565) -> ()  [unwired: 2 in, 2 out]
                        n217 = case shown="False" "OK cal3" {
                          tunnel: [0 w588] -> w564
                          frame True {
                          }
                          frame False {
                            n218 = local read "Count"() -> (w584:i32)
                            n219 = local read "SOURCE"() -> (w586:bool)
                            n220 = local read "INT"() -> (w585:i32)
                            n221 = Select(t=w584, s=w586, f=w585) -> (s? t:f=→"cal3":i32)
                            n222 = property on="cal3" class="DigNum (strict)"() -> ("NumText.BGColor"=w588:u32)  [unwired: 2 in, 2 out]
                          }
                        }
                        n223 = case shown="False" "OK cal4" {
                          tunnel: [0 w582] -> w563
                          frame True {
                          }
                          frame False {
                            n224 = local read "Count"() -> (w578:i32)
                            n225 = local read "SOURCE"() -> (w580:bool)
                            n226 = local read "INT"() -> (w579:i32)
                            n227 = property on="cal4" class="DigNum (strict)"() -> ("NumText.BGColor"=w582:u32)  [unwired: 2 in, 2 out]
                            n228 = Select(t=w578, s=w580, f=w579) -> (s? t:f=→"cal4":i32)
                          }
                        }
                        n229 = property on="cal3" class="DigNum (strict)"("NumText.TextColor"=w564) -> ()  [unwired: 2 in, 2 out]
                        n230 = case shown="True" "Manual" {
                          selector: "Manual" -> [_ w571]
                          frame False {
                          }
                          frame True {
                            n231 = Not(x=w571) -> (.not. x?=w572:bool)
                            n232 = call "Dial2.vi"() -> ("OUT"=w573:i32)
                            n233 = local write "AUTO"(w572) -> ()
                            n234 = Not Equal To 0?(x=w573) -> (x != 0?=w574:bool)
                            n235 = case shown="True" w574 {
                              tunnel: w573 -> [_ w575]
                              frame False {
                              }
                              frame True {
                                w576 = TRUE
                                n236 = local write "cal1"(w575) -> ()
                                n237 = local write "cal2"(w575) -> ()
                                n238 = local write "cal3"(w575) -> ()
                                n239 = local write "cal4"(w575) -> ()
                                n240 = local write "OK cal1"(w576) -> ()
                                n241 = local write "OK cal2"(w576) -> ()
                                n242 = local write "OK cal3"(w576) -> ()
                                n243 = local write "OK cal4"(w576) -> ()
                              }
                            }
                          }
                        }
                        n244 = property on="cal4" class="DigNum (strict)"("NumText.TextColor"=w563) -> ()  [unwired: 2 in, 2 out]
                      }
                    }
                  }
                }
              }
            }
            "GERROR" <- w439
          }
          frame #1 {
            # "256-16bit lub 1-8bit"
            # "Zapis"
            n245 = local read "Save data file"() -> (w700:bool)
            n246 = case shown="True" "FREEZE" {
              frame False {
              }
              frame True {
                n247 = flat-sequence {
                  frame #0 {
                    n248 = local read "AMP"() -> (w760:dbl)
                    n249 = local read "Hi_L"() -> (w759:dbl)
                    n250 = local read "Low_L"() -> (w758:dbl)
                    n251 = local read "INT"() -> (w757:i32)
                    n252 = local read "Count"() -> (w756:i32)
                    n253 = local read "Si[MPa]"() -> (w755:dbl)
                    n254 = local read "Quality"() -> (w754:i32)
                    n255 = local write "F Quality"(w754) -> ()
                    n256 = local write "Low_L 2"(w758) -> ()
                    n257 = local write "F Count"(w756) -> ()
                    n258 = local write "F Amp"(w760) -> ()
                    n259 = local write "Hi_L 2"(w759) -> ()
                    n260 = local write "F INT"(w757) -> ()
                    n261 = local write "F Si"(w755) -> ()
                  }
                  frame #1 {
                    w761 = FALSE ("FREEZE")
                    n262 = local write "FREEZE"(w761) -> ()
                    n263 = local write "Saveindi"(w761) -> ()
                  }
                }
              }
            }
            n264 = Array Size(array=w698) -> (size(s)=w697:i32[])
            n265 = Index Array(array=w697, index=0) -> (element=w690:i32)
            "REC." <- w690
            n266 = Decrement(x=w690) -> (x-1=w694:i32)
            n267 = Less Or Equal?(x=w690, y=0) -> (x <= y?=w689:bool)
            n268 = Select(t=FALSE, s=w689, f="DEL") -> (s? t:f=w691:bool)
            n269 = call-poly <vilib>:"Array To Matrix.vi"("Real 2D Array"=dbl[][] []) -> ("Real Matrix"=w725:T10)
            n270 = local read "File load and\nexport source"() -> (w727:string)
            n271 = case shown="True" w691 {
              tunnel: [w741 w745] -> w699
              tunnel: w698 -> [w741 w744]
              tunnel: w694 -> [_ w742]
              frame False {
              }
              frame True {
                n272 = Delete From Array(array=w744, index (row)=w742) -> (array with subset deleted=w745:dbl[][])  [unwired: 2 in, 1 out]
                n273 = local write "DEL"(FALSE ("DEL")) -> ()
              }
            }
            n274 = call-poly <vilib>:"Array To Matrix.vi"("Real 2D Array"=w699) -> ("Real Matrix"=w726:T10)
            n275 = call-poly <vilib>:"Equal.vi"("Real Matrix B"=w725, "Real Matrix A"=w726) -> ("A = B?"=w724:bool)
            n276 = Select(t=T1."Disabled and Grayed Out" ("Disabled"), s=w689, f=T1."Enabled" ("Disabled")) -> (s? t:f=w688:T1)
            n277 = Select(t=FALSE, s=w724, f=w700) -> (s? t:f=w731:bool)
            n278 = property on="DEL" class="Bool (strict)"("DisabledEnum"=w688) -> ()  [unwired: 2 in, 2 out]
            n279 = local read "GERROR"() -> (w701:bool)
            n280 = Equal?(x=w727, y="") -> (x = y?=w729:bool)
            n281 = And(x=w731, y=w729) -> (x .and. y?=w728:bool)
            n282 = case shown="True" w728 {
              frame False {
              }
              frame True {
                # "Upenienie się, że wybrano docelowe miejsce zapisu"
                n283 = local write "Save data file"(FALSE) -> ()
                n284 = call "Komunikat_OK.vi"("String 2"="Please select file save destination" ("message")) -> ()  [unwired: 1 out]
              }
            }
            n285 = Not(x=w729) -> (.not. x?=w730:bool)
            n286 = And(x=w731, y=w730) -> (x .and. y?=w702:bool)
            n287 = Or(x=w702, y=w701) -> (x .or. y?=w703:bool)
            n288 = case shown="True" w703 {
              selector: w703 -> [w764 w776]
              tunnel: w727 -> [_ w796]
              tunnel: [w764 w776] -> w704
              tunnel: w701 -> [_ w771]
              frame False {
              }
              frame True {
                w773 = "" ("y")
                w781 = "_" ("string")
                n289 = local read "Calibration file to load"() -> (w786:string)
                n290 = local read "Gain\n[dB]"() -> (w780:u8)
                n291 = Format Into String(w780) -> (resulting string=w775:string)  [unwired: 3 in, 1 out]
                n292 = Concatenate Strings(w781, "G", w775) -> (w778:string)
                n293 = Format Date/Time String(time format string (%c)="%H.%M.%S") -> (date/time string=w767:string)  [unwired: 2 in]
                n294 = Format Date/Time String(time format string (%c)="%y.%m.%d") -> (date/time string=w768:string)  [unwired: 2 in]
                n295 = Search and Replace String(case sensitive?=TRUE ("ignore case? (F)"), input string=w786, search string=".cal" ("replace string (\"\")"), replace string="") -> (result string=w779:string)  [unwired: 4 in, 3 out]
                n296 = Equal?(x=w779, y=w773) -> (x = y?=w785:bool)
                n297 = local read "Data output"() -> (w789:dbl[][])
                n298 = Select(t=w773, s=w785, f=w781) -> (s? t:f=w777:string)
                n299 = Array To Spreadsheet String(array=w789, 3:"%#5.2f" ("format string")) -> (spreadsheet string=w793:string)  [unwired: 1 in]
                n300 = Select(t="E", s=w771, f=w773) -> (s? t:f=w770:string)
                n301 = Concatenate Strings("C:\\MEB\\", w796, "\\" ("string"), w768, w781, w767, w770, w778, w777, w779, ".txt" ("string")) -> (w798:string)
                n302 = String To Path(string=w798) -> (path=w790:path)
                n303 = local write "bool_list"(TRUE ("want seconds? (F)")) -> ()
                n304 = local write "Save data file"(FALSE) -> ()
                n305 = Concatenate Strings("No.\tAMP\tHi_L\tLow_L\tINT\tCOUNT\tSi[MPa]\tQuality", "\r", w793) -> (w791:string)
                n306 = Write to Text File(file (use dialog)=w790, text=w791) -> ()  [unwired: 2 in, 3 out]
              }
            }
            n307 = Equal To 0?(x=w690) -> (x = 0?=w721:bool)
            n308 = And(x=w700, y=w721) -> (x .and. y?=w722:bool)
            n309 = case shown="True" "stop" {
              selector: "stop" -> [_ w833]
              tunnel: [FALSE w834] -> w684
              tunnel: [FALSE ("stop delay") w830] -> w685
              frame False {
              }
              frame True {
                n310 = local read "stop delay"() -> (w830:bool)
                n311 = Select(t=FALSE, s=w830, f=w833) -> (s? t:f=w832:bool)
                n312 = local write "stop"(FALSE ("stop")) -> ()
                n313 = case shown="True" w832 {
                  tunnel: [w835 w836] -> w834
                  tunnel: w830 -> [w835 _]
                  frame False {
                  }
                  frame True {
                    n314 = call "Komunikat.vi"("String 2"="This action will shut down the device.\nDo you want to continue anyway?" ("message")) -> ("OUT"=w836:bool)
                  }
                }
              }
            }
            n315 = case shown="True" w684 {
              tunnel: w685 -> [_ w849]
              frame False {
              }
              frame True {
                n316 = local read "Calibration file to load"() -> (w869:string)
                n317 = local read "THRESHOLD"() -> (w874:dbl)
                n318 = local read "Gain\n[dB]"() -> (w879:u8)
                n319 = local read "cal1"() -> (w878:dbl)
                n320 = local read "cal2"() -> (w877:dbl)
                n321 = local read "cal3"() -> (w876:dbl)
                n322 = local read "cal4"() -> (w875:dbl)
                n323 = local read "CF"() -> (w873:dbl)
                n324 = String To Byte Array(string=w869) -> (unsigned byte array=w853:u8[])
                n325 = local read "FFT RANGE"() -> (w864:cluster{"START":dbl, "END":dbl}[])
                n326 = Index Array(array=w864) -> (element #1=w863:cluster{"START":dbl, "END":dbl}, element #2=w867:cluster{"START":dbl, "END":dbl}, element #3=w866:cluster{"START":dbl, "END":dbl}, element #4=w865:cluster{"START":dbl, "END":dbl}, element #5=w846:cluster{"START":dbl, "END":dbl}, element #6=w845:cluster{"START":dbl, "END":dbl}, element #7=w844:cluster{"START":dbl, "END":dbl})  [unwired: 7 in]
                n327 = Unbundle(w863) -> ("START"=w862:dbl, "END"=w861:dbl)
                n328 = Unbundle(w867) -> ("START"=w860:dbl, "END"=w859:dbl)
                n329 = Unbundle(w866) -> ("START"=w858:dbl, "END"=w857:dbl)
                n330 = Unbundle(w865) -> ("START"=w856:dbl, "END"=w855:dbl)
                n331 = Unbundle(w846) -> ("START"=w843:dbl, "END"=w842:dbl)
                n332 = Unbundle(w845) -> ("START"=w841:dbl, "END"=w840:dbl)
                n333 = Unbundle(w844) -> ("START"=w839:dbl, "END"=w838:dbl)
                n334 = Build Array(w862, w861, w860, w859, w858, w857, w856, w855, w843, w842, w841, w840, w839, w838) -> (w852:dbl[])
                n335 = Build Array (concatenate)(w879, w878, w877, w876, w875, w874, w873, w852, w853) -> (w872:dbl[])
                n336 = call-poly <vilib>:"Write Delimited Spreadsheet.vi"("file path (dialog if empty)"=path "C:/MEBP/shift.txt", "format (%.3f)"="%.0", "1D data"=w872, "append to file? (new file:F)"=FALSE, "transpose? (no:F)"=TRUE) -> ()  [unwired: 9 in, 2 out]
                n337 = Select(t="shutdown -s -f -t 60" ("command line"), s=w849, f="shutdown -s -f -t 0" ("command line")) -> (s? t:f=w848:string)
                n338 = property on="stop" class="Bool (strict)"("DisabledEnum"=T1."Disabled and Grayed Out" ("Disabled")) -> ()  [unwired: 2 in, 2 out]
                n339 = call <vilib>:"System Exec.vi"("command line"=w848) -> ()  [unwired: 7 in, 4 out]
              }
            }
            n340 = case shown="True" w722 {
              frame False {
              }
              frame True {
                n341 = local write "Save data file"(FALSE) -> ()
                n342 = call "Komunikat_OK.vi"("String 2"="No file saved. Record list is empty." ("message")) -> ()  [unwired: 1 out]
              }
            }
            n343 = local read "F Amp"() -> (w715:dbl)
            n344 = local read "F Count"() -> (w717:dbl)
            n345 = local read "F Si"() -> (w718:dbl)
            n346 = local read "F INT"() -> (w716:dbl)
            n347 = Build Array(w715, w716, w717, w718) -> (w714:dbl[])
            n348 = Not Equal To 0?(x=w714) -> (x != 0?=w713:bool[])
            n349 = Or Array Elements(Boolean array=w713) -> (logical OR=w712:bool)
            n350 = And(x="SAVE", y=w712) -> (x .and. y?=w719:bool)
            n351 = case shown="True" w719 {
              tunnel: [w800 w803] -> w705
              tunnel: w699 -> [w800 w804]
              frame False {
              }
              frame True {
                n352 = flat-sequence {
                  tunnel: w804 -> [w816]
                  tunnel: [w814] -> w802
                  tunnel: w802 -> [w823]
                  tunnel: [w823] -> w801
                  tunnel: [w826] -> w803
                  tunnel: w801 -> [w826]
                  frame #0 {
                    w807 = nan
                    n353 = local read "REC."() -> (w811:dbl)
                    n354 = local read "F Si"() -> (w810:dbl)
                    n355 = To Long Integer(number=w810) -> (32bit integer=w806:i32)
                    n356 = To Long Integer(number=w807) -> (32bit integer=w809:i32)
                    n357 = Increment(x=w811) -> (x+1=w813:dbl)
                    n358 = Equal?(x=w806, y=w809) -> (x = y?=w808:bool)
                    n359 = Select(t=w807, s=w808, f=w806) -> (s? t:f=w805:dbl)
                    n360 = local read "F Quality"() -> (w812:dbl)
                    n361 = local read "Low_L 2"() -> (w819:dbl)
                    n362 = local read "F Count"() -> (w815:dbl)
                    n363 = local read "F Amp"() -> (w821:dbl)
                    n364 = local read "Hi_L 2"() -> (w820:dbl)
                    n365 = local read "F INT"() -> (w818:dbl)
                    n366 = Build Array(w813, w821, w820, w819, w818, w815, w805, w812) -> (w817:dbl[])
                    n367 = Insert Into Array(array=w816, index (row)=w811, new element=w817) -> (w814:dbl[][])  [unwired: 1 in]
                    "Data output" <- w814
                  }
                  frame #1 {
                    w822 = 0.0 ("F Amp")
                    n368 = local write "F Amp"(w822) -> ()
                    n369 = local write "Hi_L 2"(w822) -> ()
                    n370 = local write "Low_L 2"(w822) -> ()
                    n371 = local write "F Count"(w822) -> ()
                    n372 = local write "F Si"(w822) -> ()
                    n373 = local write "F Quality"(w822) -> ()
                    n374 = local write "F INT"(w822) -> ()
                  }
                  frame #2 {
                    n375 = local write "SAVE"(FALSE ("Add new record")) -> ()
                    "Saveindi" <- TRUE
                  }
                }
              }
            }
            n376 = local read "Gain\n[dB]"() -> (w736:u8)
            n377 = case shown="True" "AUTO" {
              frame False {
              }
              frame True {
                n378 = local read "CAL2"() -> (w748:dbl[])
                n379 = local read "Gain\n[dB]"() -> (w749:u8)
                n380 = Divide(x=w749, y=2.0) -> (x/y=w750:dbl)
                n381 = Index Array(array=w748, index=w750) -> (element=w751:dbl)
                n382 = To Long Integer(number=w751) -> (32bit integer=w746:i32)
                n383 = local write "cal1"(w746) -> ()
                n384 = local write "cal2"(w746) -> ()
                n385 = local write "cal3"(w746) -> ()
                n386 = local write "cal4"(w746) -> ()
              }
            }
            n387 = Divide(x=w736, y=u8 2) -> (x/y=w733:dbl)
            n388 = case shown="True" "Set time" {
              frame False {
              }
              frame True {
                n389 = call "TaD.vi"() -> ()  [unwired: 12 in]
              }
            }
            n390 = local read "wz"() -> (w734:u8[])
            n391 = To Unsigned Byte Integer(number=w733) -> (unsigned 8bit integer=w732:u8)
            n392 = local read "Twz"() -> (w735:refnum<k21>)
            n393 = Index Array(array=w734, index=w732) -> (element=w738:u8)
            n394 = Multiply(x=u16 256, y=w738) -> (x*y=w737:u16)
            n395 = call-poly <vilib>:"DAQmx Write.vi"("task/channels in"=w735, "data"=w737) -> ()  [unwired: 11 in, 3 out]
          }
          frame #2 {
            # "Wzorcowanie głowicy"
            n396 = case shown="True" "P_Zero" {
              frame False {
              }
              frame True {
                n397 = flat-sequence {
                  tunnel: [w888] -> w882
                  tunnel: [w896] -> w883
                  tunnel: w882 -> [w897]
                  tunnel: [w894] -> w881
                  tunnel: w883 -> [w902]
                  tunnel: w881 -> [w901]
                  frame #0 {
                    n398 = local read "Byłem"() -> (w884:bool)
                    n399 = case shown="True" w884 {
                      frame False {
                      }
                      frame True {
                        w885 = u8 0 ("Gain [dB]")
                        n400 = local write "Gain\n[dB]"(w885) -> ()
                        n401 = local write "Licznik"(w885) -> ()
                        n402 = local write "Byłem"(FALSE ("Byłem")) -> ()
                      }
                    }
                  }
                  frame #1 {
                    n403 = local read "Licznik"() -> (w887:u8)
                    n404 = Quotient & Remainder(x=w887, y=u8 2) -> (x-y*floor(x/y)=w890:u8)  [unwired: 1 out]
                    n405 = Equal To 0?(x=w890) -> (x = 0?=w888:bool)
                    n406 = case shown="True" w888 {
                      frame False {
                      }
                      frame True {
                        n407 = local read "AAZero"() -> (w891:dbl[][])
                        n408 = local read "HBN_LOOP"() -> (w892:dbl[])
                        n409 = Build Array (concatenate)(w891, w892) -> (w893:dbl[][])
                        n410 = local write "AAZero"(w893) -> ()
                      }
                    }
                  }
                  frame #2 {
                    n411 = local read "Licznik"() -> (w900:u8)
                    n412 = Increment(x=w900) -> (x+1=w898:u8)
                    n413 = local write "Licznik"(w898) -> ()
                    n414 = Greater?(x=w898, y=u8 60) -> (0:w894:bool)
                    n415 = Not(x=w894) -> (.not. x?=w895:bool)
                    n416 = And(x=w895, y=w897) -> (x .and. y?=w896:bool)
                  }
                  frame #3 {
                    n417 = case shown="True" w902 {
                      frame False {
                      }
                      frame True {
                        n418 = local read "Gain\n[dB]"() -> (w905:u8)
                        n419 = Add(x=w905, y=u8 2) -> (x+y=w904:u8)
                        n420 = local write "Gain\n[dB]"(w904) -> ()
                      }
                    }
                    n421 = case shown="True" w901 {
                      frame False {
                      }
                      frame True {
                        n422 = local write "Byłem"(TRUE ("Byłem")) -> ()
                        n423 = local read "AAZero"() -> (w911:dbl[][])
                        n424 = call-poly <vilib>:"Write Delimited Spreadsheet.vi"("file path (dialog if empty)"=path "C:/MEBP/pzero.txt", "format (%.3f)"="%.4f", "2D data"=w911, "append to file? (new file:F)"=FALSE, "transpose? (no:F)"=FALSE) -> ()  [unwired: 9 in, 2 out]
                        n425 = local write "P_Zero"(FALSE ("P_Zero")) -> ()
                      }
                    }
                  }
                }
              }
            }
          }
          frame #3 {
            # "Autoshutdown"
            # "Kontrola ładowania"
            n426 = local read "BAT"() -> (w935:refnum<k21>)
            n427 = call-poly <vilib>:"DAQmx Read.vi"("task/channels in"=w935) -> ("data"=w934:dbl)  [unwired: 12 in, 2 out]
            n428 = Multiply(x=2.0, y=w934) -> (x*y=w917:dbl)
            n429 = local read "OK"() -> (w931:bool)
            n430 = feedback #2() -> (w921:dbl[])  [unwired: 1 in]
            n431 = feedback #3() -> (w919:bool)  [unwired: 1 in]
            n432 = Select(t=dbl[] [], s=w919, f=w921) -> (s? t:f=w920:dbl[])
            n433 = Build Array (concatenate)(w920, w917) -> (w925:dbl[])
            n434 = feedback-in #2(w925) -> ()
            n435 = Not(x=w931) -> (.not. x?=w930:bool)
            n436 = Add Array Elements(numeric array=w925) -> (sum=w927:dbl)
            n437 = Array Size(array=w925) -> (size(s)=w924:i32)
            n438 = Divide(x=w927, y=3.0) -> (x/y=w913:dbl)
            n439 = Equal?(x=w924, y=3) -> (x = y?=w918:bool)
            n440 = feedback-in #3(w918) -> ()
            n441 = Add(x=w913, y=0.6) -> (x+y=w914:dbl)
            n442 = case shown="True" w918 {
              tunnel: w914 -> [_ w938]
              tunnel: [FALSE w937] -> w916
              frame False {
              }
              frame True {
                n443 = Less Or Equal?(x=w938, y=14.9) -> (x <= y?=→"Bat_Low":bool)
                n444 = Less Or Equal?(x=w938, y=14.6) -> (x <= y?=w937:bool)
                "Supply [V]" <- w938
              }
            }
            n445 = And(x=w916, y=TRUE) -> (x .and. y?=w929:bool)
            n446 = And(x=w929, y=w930) -> (x .and. y?=w932:bool)
            n447 = case shown="True" w932 {
              selector: w932 -> [_ w942]
              frame False {
                (unwired) FALSE ("Time has Elapsed")
              }
              frame True {
                n448 = local write "stop"(w942) -> ()
                n449 = local write "stop delay"(w942) -> ()
                n450 = call "Komunikat_OK.vi"("String 2"="Battery Low\nAuto Power OFF in 60s" ("Message")) -> ("OUT"=→"OK":bool)
              }
            }
          }
        }
        n451 = local read "Bat_Low"() -> (w135:bool)
        n452 = property on="Tab Control" class="TabCtl (strict)"("MultColors"=TRUE ("Allow Multiple Colors")) -> ("Pages"=w143:refnum<vi>[])  [unwired: 2 in, 2 out]
        n453 = case shown="True" w135 {
          tunnel: [u32 744192 u32 16742513] -> w136
          frame False {
          }
          frame True {
          }
        }
        n454 = Index Array(array=w143, index="Tab Control") -> (element=w134:refnum<vi>)
        n455 = Delete From Array(array=w143, index="Tab Control") -> (array with subset deleted=w141:refnum<vi>[])  [unwired: 1 in, 1 out]
        n456 = Select(t=dbl[][] [], s=w129, f=w130) -> (s? t:f=w146:dbl[][])
        n457 = Index Array(array=w141) -> (element #1=w140:refnum<vi>, element #2=w139:refnum<vi>, element #3=w138:refnum<vi>, element #4=w137:refnum<vi>)  [unwired: 4 in]
        n458 = property class="Page"(reference=w134, "FG Color"=u32 0 ("Colors:FG Color")) -> ()  [unwired: 1 in, 2 out]
        n459 = property class="Page"(reference=w134, "BG Color"=u32 16448250 ("Colors:BG Color")) -> ()  [unwired: 1 in, 2 out]
        n460 = property class="Page"(reference=w140, "FG Color"=w136) -> ()  [unwired: 1 in, 2 out]
        n461 = property class="Page"(reference=w139, "FG Color"=w136) -> ()  [unwired: 1 in, 2 out]
        n462 = property class="Page"(reference=w138, "FG Color"=w136) -> ()  [unwired: 1 in, 2 out]
        n463 = property class="Page"(reference=w137, "FG Color"=w136) -> ()  [unwired: 1 in, 2 out]
        n464 = case shown="\"STOR\"" "Tab Control" {
          frame "STAT", Default {
            n465 = local write "Pomiar_main"(TRUE ("Pomiar_main")) -> ()
          }
          frame "MEAS" {
            w151 = TRUE ("Oblicz")
            n466 = local read "Saveindi"() -> (w152:bool)
            n467 = case shown="True" w152 {
              frame False {
                n468 = property on="SAVE" class="Bool (strict)"("DisabledEnum"=T1."Enabled" ("Disabled")) -> ()  [unwired: 2 in, 2 out]
              }
              frame True {
                n469 = property on="SAVE" class="Bool (strict)"("DisabledEnum"=T1."Disabled and Grayed Out" ("Disabled")) -> ()  [unwired: 2 in, 2 out]
              }
            }
            n470 = local write "Pomiar_main"(w151) -> ()
            n471 = local write "Oblicz"(w151) -> ()
          }
          frame "CAL" {
            w155 = TRUE
            n472 = local read "Load calibration"() -> (w160:bool)
            n473 = local read "Import calibration files"() -> (w161:bool)
            n474 = List Folder(path=path "C:/MEB", pattern="*.cal") -> (filenames=w159:string[])  [unwired: 2 in, 3 out]
            n475 = property on="Calibration file to load" class="CmbBox"("Strings[]"=w159) -> ()  [unwired: 2 in, 2 out]
            n476 = case shown="True" w160 {
              frame False {
              }
              frame True {
                w205 = T3 0 items=["no dialog", "OK message", "continue or stop message", "OK message + warnings", "continue/stop + warnings"] ("type of dialog (OK msg:1)")
                w215 = T3 0 items=["no dialog", "OK message", "continue or stop message", "OK message + warnings", "continue/stop + warnings"] ("type of dialog (OK msg:1)")
                n477 = First Call?() -> (First Call?: T/F=w213:bool)
                n478 = local write "Load calibration"(FALSE ("Cal_initialize")) -> ()
                n479 = case shown="True" w213 {
                  tunnel: ["err" ("string") w231] -> w212
                  frame False {
                  }
                  frame True {
                    n480 = call-poly <vilib>:"Read Delimited Spreadsheet.vi"("file path (dialog if empty)"=path "C:/MEBP/shift.txt", "transpose? (F)"=TRUE) -> ("first row"=w230:dbl[])  [unwired: 8 in, 5 out]
                    n481 = Array Subset(array=w230, index=21) -> (w229:dbl[])  [unwired: 1 in]
                    n482 = Byte Array To String(unsigned byte array=w229) -> (string=w231:string)
                  }
                }
                n483 = Select(t=w212, s=w213, f="Calibration file to load") -> (s? t:f=w211:string)
                n484 = Concatenate Strings("C:\\MEB\\", w211) -> (w210:string)
                n485 = String To Path(string=w210) -> (path=w217:path)
                n486 = Concatenate Strings(w210, "2" ("string")) -> (w208:string)
                n487 = property on="Calibration file to load" class="CmbBox"("Value"=w211) -> ()  [unwired: 2 in, 2 out]
                n488 = String To Path(string=w208) -> (path=w207:path)
                n489 = call-poly <vilib>:"Read Delimited Spreadsheet.vi"("file path (dialog if empty)"=w217, "transpose? (F)"=TRUE) -> ("all rows"=w222:dbl[][], "error out"=w216:errorcluster)  [unwired: 8 in, 4 out]
                "CAL" <- w222
                n490 = call-poly <vilib>:"Read Delimited Spreadsheet.vi"("file path (dialog if empty)"=w207) -> ("all rows"=w204:dbl[][], "error out"=w206:errorcluster)  [unwired: 9 in, 4 out]
                n491 = Index Array(array=w222) -> (element #1=w221:dbl[], element #2=w220:dbl[])  [unwired: 4 in]
                "XX" <- w221
                "YY" <- w220
                n492 = call <vilib>:"Simple Error Handler.vi"("type of dialog (OK msg:1)"=w215, "error in (no error)"=w216) -> ()  [unwired: 3 in, 5 out]
                n493 = call <vilib>:"Simple Error Handler.vi"("type of dialog (OK msg:1)"=w205, "error in (no error)"=w206) -> ("error?"=w198:bool)  [unwired: 3 in, 4 out]
                n494 = case shown="True" w198 {
                  frame False {
                  }
                  frame True {
                    n495 = call "Komunikat_OK.vi"("String 2"="There is no ZERO POINT associated file." ("error source (\" \")")) -> ()  [unwired: 1 out]
                  }
                }
                n496 = Select(t=T1."Disabled and Grayed Out" ("Disabled"), s=w198, f=T1."Enabled" ("Disabled")) -> (s? t:f=w201:T1)
                n497 = property on="AUTO" class="Bool (strict)"("DisabledEnum"=w201) -> ()  [unwired: 2 in, 2 out]
                n498 = Index Array(array=w204, index (col)=0 ("disabled index (col)")) -> (element=→"CAL2":dbl[])  [unwired: 1 in]
                n499 = Build Cluster Array(w221, w220) -> (→"XY Graph":cluster{"Numeric":dbl, "Numeric":dbl}[])
              }
            }
            n500 = case shown="True" "Delete cal file" {
              frame False {
              }
              frame True {
                n501 = local read "Calibration file to load"() -> (w166:string)
                n502 = Concatenate Strings("C:\\MEB\\", w166) -> (w168:string)
                n503 = String To Path(string=w168) -> (path=w164:path)
                n504 = call "Komunikat.vi"("String 2"="Are you sure you want to delete\nthis calibration file?" ("prompt (Delete)")) -> ("OUT"=w162:bool)
                n505 = case shown="True" w162 {
                  selector: w162 -> [w169 _]
                  tunnel: w164 -> [_ w172]
                  tunnel: [w169 w171] -> w163
                  frame False {
                  }
                  frame True {
                    w173 = T3 0 items=["no dialog", "OK message", "continue or stop message", "OK message + warnings", "continue/stop + warnings"] ("type of dialog (OK msg:1)")
                    n506 = Delete(path (use dialog)=w172) -> (cancelled=w171:bool, error out=w170:errorcluster)  [unwired: 4 in, 1 out]
                    n507 = call <vilib>:"Simple Error Handler.vi"("type of dialog (OK msg:1)"=w173, "error in (no error)"=w170) -> ()  [unwired: 3 in, 5 out]
                  }
                }
                n508 = case shown="False" w163 {
                  frame False {
                    n509 = property on="Calibration file to load" class="CmbBox"() -> ("Strings[]"=w175:string[])  [unwired: 2 in, 2 out]
                    n510 = Index Array(array=w175, index=0) -> (element=w176:string)
                    n511 = property on="Calibration file to load" class="CmbBox"("Value"=w176) -> ()  [unwired: 2 in, 2 out]
                  }
                  frame True {
                  }
                }
              }
            }
            n512 = case shown="True" w161 {
              frame False {
              }
              frame True {
                w185 = path "D:/MEB" ("source path")
                w188 = T3 0 items=["no dialog", "OK message", "continue or stop message", "OK message + warnings", "continue/stop + warnings"] ("type of dialog (OK msg:1)")
                n513 = local write "Import calibration files"(FALSE ("Replace calibration files")) -> ()
                n514 = Path To String(path=w185) -> (string=w186:string)
                n515 = List Folder(path=w185, pattern="*.cal*") -> (filenames=w187:string[], error out=w177:errorcluster)  [unwired: 2 in, 2 out]
                n516 = for {
                  tunnel: w187 -> [w195] mode=indexing
                  tunnel: w186 -> [w196]
                  tunnel: [w191] -> w183 mode=indexing
                  n517 = Concatenate Strings(w196, "\\" ("string"), w195) -> (w193:string)
                  n518 = String To Path(string=w193) -> (path=w192:path)
                  n519 = Copy(9:TRUE ("overwrite (F)"), 10:path "C:/MEB" ("target path (use dialog)"), 11:w192) -> (0:w191:errorcluster)  [unwired: 2 in, 2 out]
                }
                n520 = Merge Errors(w183, w177) -> (w182:errorcluster)
                n521 = call <vilib>:"Simple Error Handler.vi"("type of dialog (OK msg:1)"=w188, "error in (no error)"=w182) -> ("error?"=w179:bool)  [unwired: 3 in, 4 out]
                n522 = Select(t="File not found.\nFiles with *.cal or *.cal2 extension should be located on external drive in folder ..\\MEB.", s=w179, f="Import successfull.") -> (s? t:f=w178:string)
                n523 = call "Komunikat_OK.vi"("String 2"=w178) -> ()  [unwired: 1 out]
              }
            }
            n524 = local write "Pomiar_main"(w155) -> ()
            n525 = local write "Oblicz"(w155) -> ()
          }
          frame "STOR" {
            n526 = flat-sequence {
              frame #0 {
                w252 = 0 ("y")
                w262 = FALSE
                w283 = T3 0 items=["no dialog", "OK message", "continue or stop message", "OK message + warnings", "continue/stop + warnings"] ("type of dialog (OK msg:1)")
                # "T<0?\nY:T=0\nN:T\nOut:T"
                # "Save data file lead to T=L-N and V=L-1"
                # "V>L-1?\nY:V=L-1\nN:V\nOut:V"
                # "V<0?\nY:V=0\nN:V\nOut:V"
                # "V<=T?\nY:T-1\nN:T\nOut:T"
                # "Up or down"
                # "V>=T+N-1?\nY:T+1\nN:T\nOut:T"
                n527 = local read "File load and\nexport source"() -> (w285:string)
                n528 = property on="Listbox" class="LstBox (strict)"("Scrollbar Visible"=FALSE ("Visible Items:Vertical Scrollbar Visible")) -> ("Value"=w257:i32, "Number of Rows"=w241:u32, "Top Row"=w256:i32)  [unwired: 2 in, 2 out]
                n529 = local read "Export to drive"() -> (w286:bool)
                n530 = local write "Oblicz"(w262) -> ()
                n531 = local write "Pomiar_main"(w262) -> ()
                n532 = local read "bool_list"() -> (w248:bool)
                n533 = To Long Integer(number=w241) -> (32bit integer=w242:i32)
                n534 = Or(x="ListuDow", y="ListUP") -> (x .or. y?=w260:bool)
                n535 = Equal?(x=w285, y="") -> (x = y?=w291:bool)
                n536 = And(x=w286, y=w291) -> (x .and. y?=w266:bool)
                n537 = case shown="True" w266 {
                  frame False {
                  }
                  frame True {
                    n538 = call "Komunikat_OK.vi"("String 2"="Please select export source." ("message")) -> ()  [unwired: 1 out]
                  }
                }
                n539 = Not(x=w291) -> (.not. x?=w292:bool)
                n540 = case shown="True" w260 {
                  tunnel: "ListUP" -> [_ w331]
                  tunnel: [0 w328] -> w258
                  frame False {
                  }
                  frame True {
                    n541 = Select(t=-1, s=w331, f=1) -> (s? t:f=w328:i32)
                  }
                }
                n542 = Concatenate Strings("C:\\MEB\\", w285, "\\" ("string")) -> (w276:string)
                n543 = And(x=w286, y=w292) -> (x .and. y?=w293:bool)
                n544 = String To Path(string=w276) -> (path=w294:path)
                n545 = case shown="True" w293 {
                  selector: w293 -> [_ w376]
                  tunnel: w285 -> [_ w396]
                  tunnel: w291 -> [_ _]
                  frame False {
                  }
                  frame True {
                    w377 = TRUE ("run minimized? (F)")
                    w382 = "0x00000057" ("regular expression")
                    w395 = "0x00000002" ("regular expression")
                    w394 = "0x00000003" ("regular expression")
                    w393 = "0x00000013" ("regular expression")
                    # "Dopasowanie kodu do opisu błędu"
                    # "Opis błędów"
                    # "Wybór błędu"
                    # "Wykryta nazwa błędu"
                    # "Stworzenie arraya błędów"
                    # "Not enough space"
                    # "No device connected"
                    # "Device removed too early"
                    n546 = local write "Export in\nprogress"(w376) -> ()
                    n547 = Concatenate Strings("robocopy C:\\MEB\\", w396, " D:\\MEB\\", w396, " /E /R:0", "\r\n") -> (w397:string)
                    n548 = call <vilib>:"System Exec.vi"("run minimized? (F)"=w377, "wait until completion? (T)"=w377, "working directory"=path "c:/", "standard input"=w397, "command line"="cmd") -> ("standard output"=w383:string)  [unwired: 3 in, 3 out]
                    n549 = Match Pattern(string=w383, regular expression=w393) -> (match substring=w404:string)  [unwired: 1 in, 3 out]
                    n550 = Match Pattern(string=w383, regular expression=w394) -> (match substring=w403:string)  [unwired: 1 in, 3 out]
                    n551 = Match Pattern(string=w404, regular expression=w395) -> (match substring=w402:string)  [unwired: 1 in, 3 out]
                    n552 = Match Pattern(string=w383, regular expression=w382) -> (match substring=w384:string)  [unwired: 1 in, 3 out]
                    n553 = Build Array(w395, w394, w393, w382, "") -> (w392:string[])
                    n554 = Concatenate Strings(w404, w403, w402, w384, "") -> (w391:string)
                    n555 = Build Array("File export error. Device removed too early.", "File export error. No device connected.", "File export error. Try again.", "File export error. Not enough space on disc to complete.", "Files exported successfully.") -> (w387:string[])
                    n556 = Search 1D Array(1D array=w392, element=w391) -> (index of element=w386:i32)  [unwired: 1 in]
                    n557 = Index Array(array=w387, index=w386) -> (element=w381:string)
                    n558 = local write "Export to drive"(FALSE ("Export to drive")) -> ()
                    n559 = call "Komunikat_OK.vi"("String 2"=w381) -> ()  [unwired: 1 out]
                  }
                }
                n560 = List Folder(path=w294) -> (filenames=w265:string[], error out=w284:errorcluster)  [unwired: 3 in, 2 out]
                n561 = Add(x=w257, y=w258) -> (x+y=w255:i32)
                n562 = for {
                  tunnel: w265 -> [w334] mode=indexing
                  tunnel: [w332] -> w264 mode=indexing
                  n563 = Search and Replace String(input string=w334, search string=".txt" ("substring (\"\")")) -> (result string=w332:string)  [unwired: 6 in, 3 out]
                }
                n564 = in-place {
                  in-place-border: w255 -> [w316]
                  in-place-border: [w315] -> w254
                  w317 = 0 ("y")
                  n565 = Less?(x=w316, y=w317) -> (x < y?=w318:bool)
                  n566 = Select(t=w317, s=w318, f=w316) -> (s? t:f=w315:i32)
                }
                n567 = local read "Delete folder content"() -> (w267:bool)
                n568 = local read "Delete content"() -> (w240:bool)
                n569 = call <vilib>:"Simple Error Handler.vi"("type of dialog (OK msg:1)"=w283, "error in (no error)"=w284) -> ()  [unwired: 3 in, 5 out]
                n570 = property on="Listbox" class="LstBox (strict)"("Item Names"=w264) -> ()  [unwired: 2 in, 2 out]
                n571 = Equal?(x="Listbox", y=-1) -> (x = y?=w274:bool)
                n572 = local read "Preview data"() -> (w279:bool)
                n573 = Select(t=0, s=w274, f="Listbox") -> (s? t:f=w272:i32)
                n574 = Array Size(array=w265) -> (size(s)=w251:i32)
                n575 = Not Equal To 0?(x=w251) -> (x != 0?=w238:bool)
                n576 = Decrement(x=w251) -> (x-1=w247:i32)
                n577 = And(x=w267, y=w238) -> (x .and. y?=w239:bool)
                n578 = in-place {
                  in-place-border: [w309] -> w250
                  in-place-border: w254 -> [w307]
                  in-place-border: w247 -> [w306]
                  n579 = Greater?(x=w307, y=w306) -> (0:w308:bool)
                  n580 = Select(t=w306, s=w308, f=w307) -> (s? t:f=w309:i32)
                }
                n581 = in-place {
                  in-place-border: w256 -> [w322]
                  in-place-border: w242 -> [w323]
                  in-place-border: w250 -> [w321]
                  in-place-border: [w319] -> w243
                  n582 = Increment(x=w322) -> (x+1=w320:i32)
                  n583 = Add(x=w322, y=w323) -> (x+y=w324:i32)
                  n584 = Decrement(x=w324) -> (x-1=w325:i32)
                  n585 = Greater Or Equal?(x=w321, y=w325) -> (x >= y?=w326:bool)
                  n586 = Select(t=w320, s=w326, f=w322) -> (s? t:f=w319:i32)
                }
                n587 = case shown="True" w239 {
                  tunnel: w265 -> [_ w353]
                  tunnel: w276 -> [_ w352]
                  frame False {
                  }
                  frame True {
                    n588 = local write "Delete folder content"(FALSE ("Delete content")) -> ()
                    n589 = call "Komunikat.vi"("String 2"="This will delete all content in the folder.\nDo you still want to continue?") -> ("OUT"=w350:bool)
                    n590 = case shown="True" w350 {
                      tunnel: w353 -> [_ w355]
                      tunnel: w352 -> [_ w354]
                      frame False {
                      }
                      frame True {
                        n591 = for {
                          tunnel: w355 -> [w362] mode=indexing
                          tunnel: w354 -> [w359]
                          w358 = T3 0 items=["no dialog", "OK message", "continue or stop message", "OK message + warnings", "continue/stop + warnings"] ("type of dialog (OK msg:1)")
                          n592 = Concatenate Strings(w359, w362) -> (w361:string)
                          n593 = String To Path(string=w361) -> (path=w360:path)
                          n594 = Delete(path (use dialog)=w360) -> (error out=w356:errorcluster)  [unwired: 4 in, 2 out]
                          n595 = call <vilib>:"Simple Error Handler.vi"("error code (no error:0)"=0, "type of dialog (OK msg:1)"=w358, "error in (no error)"=w356) -> ()  [unwired: 2 in, 5 out]
                        }
                      }
                    }
                  }
                }
                n596 = Index Array(array=w265, index=w272) -> (element=w269:string)
                n597 = Not Equal?(x=w269, y="") -> (x != y?=w236:bool)
                n598 = Select(t=T1."Enabled" ("Disabled"), s=w236, f=T1."Disabled and Grayed Out" ("Disabled")) -> (s? t:f=w235:T1)
                n599 = property on="Delete folder content" class="Bool (strict)"("DisabledEnum"=w235) -> ()  [unwired: 2 in, 2 out]
                n600 = property on="Delete content" class="Bool (strict)"("DisabledEnum"=w235) -> ()  [unwired: 2 in, 2 out]
                n601 = And(x=w240, y=w236) -> (x .and. y?=w237:bool)
                n602 = in-place {
                  in-place-border: w250 -> [w313]
                  in-place-border: w243 -> [w311]
                  in-place-border: [w312] -> w244
                  in-place-border: [w311] -> _
                  n603 = Decrement(x=w311) -> (x-1=w310:i32)
                  n604 = Less Or Equal?(x=w313, y=w311) -> (x <= y?=w314:bool)
                  n605 = Select(t=w310, s=w314, f=w311) -> (s? t:f=w312:i32)
                }
                n606 = Not Equal To 0?(x=w251) -> (x != 0?=w281:bool)
                n607 = Concatenate Strings(w276, w269) -> (w288:string)
                n608 = case shown="True" w237 {
                  tunnel: w269 -> [_ w337]
                  tunnel: w276 -> [_ w336]
                  frame False {
                  }
                  frame True {
                    n609 = local write "Delete content"(FALSE ("Delete content single")) -> ()
                    n610 = call "Komunikat.vi"("String 2"="This will delete the selected file.\nDo you still want to continue?") -> ("OUT"=w338:bool)
                    n611 = case shown="True" w338 {
                      tunnel: w337 -> [_ w344]
                      tunnel: w336 -> [_ w343]
                      frame False {
                      }
                      frame True {
                        w340 = T3 0 items=["no dialog", "OK message", "continue or stop message", "OK message + warnings", "continue/stop + warnings"] ("type of dialog (OK msg:1)")
                        n612 = Concatenate Strings(w343, w344) -> (w345:string)
                        n613 = String To Path(string=w345) -> (path=w346:path)
                        n614 = Delete(path (use dialog)=w346) -> (error out=w342:errorcluster)  [unwired: 4 in, 2 out]
                        n615 = call <vilib>:"Simple Error Handler.vi"("error code (no error:0)"=0, "type of dialog (OK msg:1)"=w340, "error in (no error)"=w342) -> ()  [unwired: 2 in, 5 out]
                      }
                    }
                  }
                }
                n616 = And(x=w279, y=w281) -> (x .and. y?=w282:bool)
                n617 = String To Path(string=w288) -> (path=w287:path)
                n618 = Not(x=w281) -> (.not. x?=w280:bool)
                n619 = And(x=w279, y=w280) -> (x .and. y?=w278:bool)
                n620 = case shown="True" w282 {
                  tunnel: w287 -> [_ w373]
                  tunnel: w269 -> [_ w371]
                  frame False {
                  }
                  frame True {
                    n621 = call-poly <vilib>:"Read Delimited Spreadsheet.vi"("file path (dialog if empty)"=w373, "transpose? (F)"=TRUE) -> ("all rows"=w365:dbl[][])  [unwired: 8 in, 5 out]
                    n622 = Transpose 2D Array(2D array=w365) -> (transposed array=w364:dbl[][])
                    n623 = Increment(x="Plot selection") -> (x+1=w366:u16)
                    n624 = local write "Preview data"(FALSE ("Export to drive")) -> ()
                    n625 = Index Array(array=w364, index (col)=w366) -> (element=w370:dbl[])  [unwired: 1 in]
                    n626 = Array Subset(array=w370, index=1) -> (→"Preview":dbl[])  [unwired: 1 in]
                    "Active file" <- w371
                  }
                }
                n627 = in-place {
                  in-place-border: [w305] -> w245
                  in-place-border: w251 -> [w304]
                  in-place-border: w242 -> [w303]
                  in-place-border: w250 -> [w300]
                  in-place-border: [w299] -> w249
                  in-place-border: w248 -> [w298]
                  in-place-border: w247 -> [w297]
                  in-place-border: w244 -> [w296]
                  n628 = Subtract(x=w304, y=w303) -> (x-y=w302:i32)
                  n629 = Select(t=w297, s=w298, f=w300) -> (s? t:f=w299:i32)
                  n630 = Increment(x=w302) -> (x+1=w301:i32)
                  n631 = Select(t=w301, s=w298, f=w296) -> (s? t:f=w305:i32)
                }
                n632 = case shown="True" w278 {
                  frame False {
                  }
                  frame True {
                    n633 = local write "Preview data"(FALSE ("Export to drive")) -> ()
                    n634 = call "Komunikat_OK.vi"("String 2"="No files to show." ("message")) -> ()  [unwired: 1 out]
                  }
                }
                n635 = Less?(x=w245, y=w252) -> (x < y?=w253:bool)
                n636 = Select(t=w252, s=w253, f=w245) -> (s? t:f=w246:i32)
                n637 = property on="Listbox" class="LstBox (strict)"("Value"=w249, "Active Row"=w249, "Top Row"=w246) -> ()  [unwired: 2 in, 2 out]
                n638 = case shown="True" w248 {
                  frame False {
                  }
                  frame True {
                    n639 = local write "bool_list"(FALSE) -> ()
                  }
                }
                "Export in\nprogress" <- FALSE ("Exporting files")
              }
            }
          }
          frame "TOOL" {
            w409 = cluster{u32, u32} {16777216, 16777216}
            n640 = local read "Update"() -> (w407:bool)
            n641 = local write "Pomiar_main"(TRUE) -> ()
            n642 = case shown="True" w407 {
              frame False {
              }
              frame True {
                n643 = flat-sequence {
                  frame #0 {
                    n644 = local read "enUP"() -> (w413:dbl)
                    n645 = Increment(x=w413) -> (x+1=w412:dbl)
                    "enUP" <- w412
                    n646 = Equal?(x=w412, y=5.0) -> (x = y?=w414:bool)
                    n647 = Greater Or Equal?(x=w412, y=1.0) -> (x >= y?=→"Boolean 5":bool)
                    n648 = Greater Or Equal?(x=w412, y=2.0) -> (x >= y?=→"Boolean 6":bool)
                    n649 = Greater Or Equal?(x=w412, y=3.0) -> (x >= y?=→"Boolean 7":bool)
                    n650 = Greater Or Equal?(x=w412, y=4.0) -> (x >= y?=→"Boolean 8":bool)
                    n651 = case shown="True" w414 {
                      frame False {
                      }
                      frame True {
                        w424 = T3 0 items=["no dialog", "OK message", "continue or stop message", "OK message + warnings", "continue/stop + warnings"] ("type of dialog (OK msg:1)")
                        w433 = FALSE
                        n652 = local write "enUP"(0.0 ("x+1")) -> ()
                        n653 = local write "Boolean 5"(w433) -> ()
                        n654 = local write "Boolean 6"(w433) -> ()
                        n655 = local write "Boolean 7"(w433) -> ()
                        n656 = local write "Boolean 8"(w433) -> ()
                        n657 = List Folder(path=path "D:/MEBU") -> (filenames=w431:string[], error out=w426:errorcluster)  [unwired: 3 in, 2 out]
                        n658 = Search 1D Array(1D array=w431, element="MEB2CXu.exe") -> (index of element=w429:i32)  [unwired: 1 in]
                        n659 = call <vilib>:"Simple Error Handler.vi"("error code (no error:0)"=0, "type of dialog (OK msg:1)"=w424, "error in (no error)"=w426) -> ()  [unwired: 2 in, 5 out]
                        n660 = Not Equal?(x=w429, y=-1) -> (x != y?=w427:bool)
                        n661 = case shown="True" w427 {
                          frame False {
                          }
                          frame True {
                            w436 = TRUE ("wait until completion? (T)")
                            n662 = call <vilib>:"System Exec.vi"("run minimized? (F)"=w436, "wait until completion? (T)"=w436, "working directory"=path "C:/MEBP", "command line"="cmd /c updater.exe" ("standard input")) -> ()  [unwired: 4 in, 4 out]
                          }
                        }
                      }
                    }
                  }
                  frame #1 {
                    n663 = local write "Update"(FALSE ("Update")) -> ()
                  }
                }
              }
            }
            n664 = Build Array(w409, w409, w409, w409, w409, w409) -> (w410:cluster{u32, u32}[])
            n665 = property on="Update" class="Bool (strict)"("Colors [4]"=w410) -> ()  [unwired: 2 in, 2 out]
            n666 = local write "Oblicz"(TRUE ("Oblicz")) -> ()
          }
        }
      }
    }
  }
